vi "PropertyEditor.vi"(7 "Popup? (F)":bool, 8 "error in (no error)":errorcluster, 11 "Component in":refnum<class "IComponent.lvclass">) -> (0 "error out":errorcluster)   [LabVIEW 2022 SP3, in "Property Editor.lvlib"]
uses:
  <instrlib>/openDAQ/Examples/Property Editor/Property Editor.lvlib
  <instrlib>/openDAQ/Public/Classes/IComponent/IComponent.lvclass
  C:/Program Files (x86)/National Instruments/LabVIEW 2022/instr.lib/openDAQ/Public/Classes/IBaseObject/IBaseObject.lvclass
  C:/Program Files (x86)/National Instruments/LabVIEW 2022/instr.lib/openDAQ/Public/Classes/IPropertyObject/IPropertyObject.lvclass
  <instrlib>/openDAQ/Examples/Property Editor/TypeDef/State.ctl
  <instrlib>/openDAQ/Examples/Property Editor/TypeDef/Context.ctl
  <instrlib>/openDAQ/Public/Classes/IProperty/IProperty.lvclass
  <instrlib>/openDAQ/Examples/Property Editor/TypeDef/DisplayType.ctl
  <vilib>/picture/picture.llb/imagedata.ctl
  <vilib>/Utility/miscctls.llb/LVComboBoxStrsAndValuesArrayTypeDef.ctl
  <instrlib>/openDAQ/Public/Classes/IBaseObject/IBaseObject.lvclass/IBaseObject.ctl
  <instrlib>/openDAQ/Public/Classes/IBaseObject/Accessor/Read reference.vi
  <vilib>/Utility/error.llb/Trim Whitespace One-Sided.vi
  <instrlib>/openDAQ/Public/Classes/IInstance/IInstance.lvclass
  C:/Program Files (x86)/National Instruments/LabVIEW 2022/instr.lib/openDAQ/Public/Classes/IComponent/IComponent.lvclass
  <instrlib>/openDAQ/Public/Classes/IDevice/IDevice.lvclass
  <instrlib>/openDAQ/Public/Classes/daqCoreTypes/IFloat/IFloat.lvclass
  <instrlib>/openDAQ/Public/Classes/daqCoreTypes/IInteger/IInteger.lvclass
  <instrlib>/openDAQ/Public/Classes/daqCoreTypes/IBoolean/IBoolean.lvclass
  <instrlib>/openDAQ/Public/Classes/daqCoreTypes/IString/IString.lvclass
  <instrlib>/openDAQ/Public/Classes/daqCoreTypes/IRatio/IRatio.lvclass
  <instrlib>/openDAQ/Public/Classes/daqCoreTypes/IList/IList.lvclass
  <instrlib>/openDAQ/Public/Classes/IBaseObject/Polymorphic/borrowInterface/borrowListInterface.vi
  <instrlib>/openDAQ/Public/Classes/daqCoreTypes/IList/Polymorphic/getList/getStringList.vi
  <instrlib>/openDAQ/Public/Classes/daqCoreTypes/IList/Polymorphic/getList/getFloatList.vi
  <instrlib>/openDAQ/Public/Classes/daqCoreTypes/IList/Polymorphic/getList/getIntegerList.vi
  <instrlib>/openDAQ/Public/Classes/IBaseObject/Polymorphic/borrowInterface/borrowDictInterface.vi
  <instrlib>/openDAQ/Public/Classes/daqCoreTypes/IDict/Polymorphic/getValueList/getIntegerValueList.vi
  <instrlib>/openDAQ/Public/Classes/daqCoreTypes/IDict/Polymorphic/getValueList/getFloatValueList.vi
  <instrlib>/openDAQ/Public/Classes/daqCoreTypes/IDict/Polymorphic/getValueList/getStringValueList.vi
  <instrlib>/openDAQ/Public/Classes/IBaseObject/IBaseObject.lvclass
  <instrlib>/openDAQ/Public/Classes/daqUtils/daqUtils.lvlib
  <instrlib>/openDAQ/Public/Classes/daqCoreTypes/IDict/IDict.lvclass
panel:
  in  "btn:PropertyRefresh":bool
  in  "Btn:Stop":bool
  in  "RB:Selector":T1(radio)
  in  "Tree.Components":string(tree)="Devices"
  in  "Tree.Properties":string(tree)
  in  "Selection Values":string(combo)
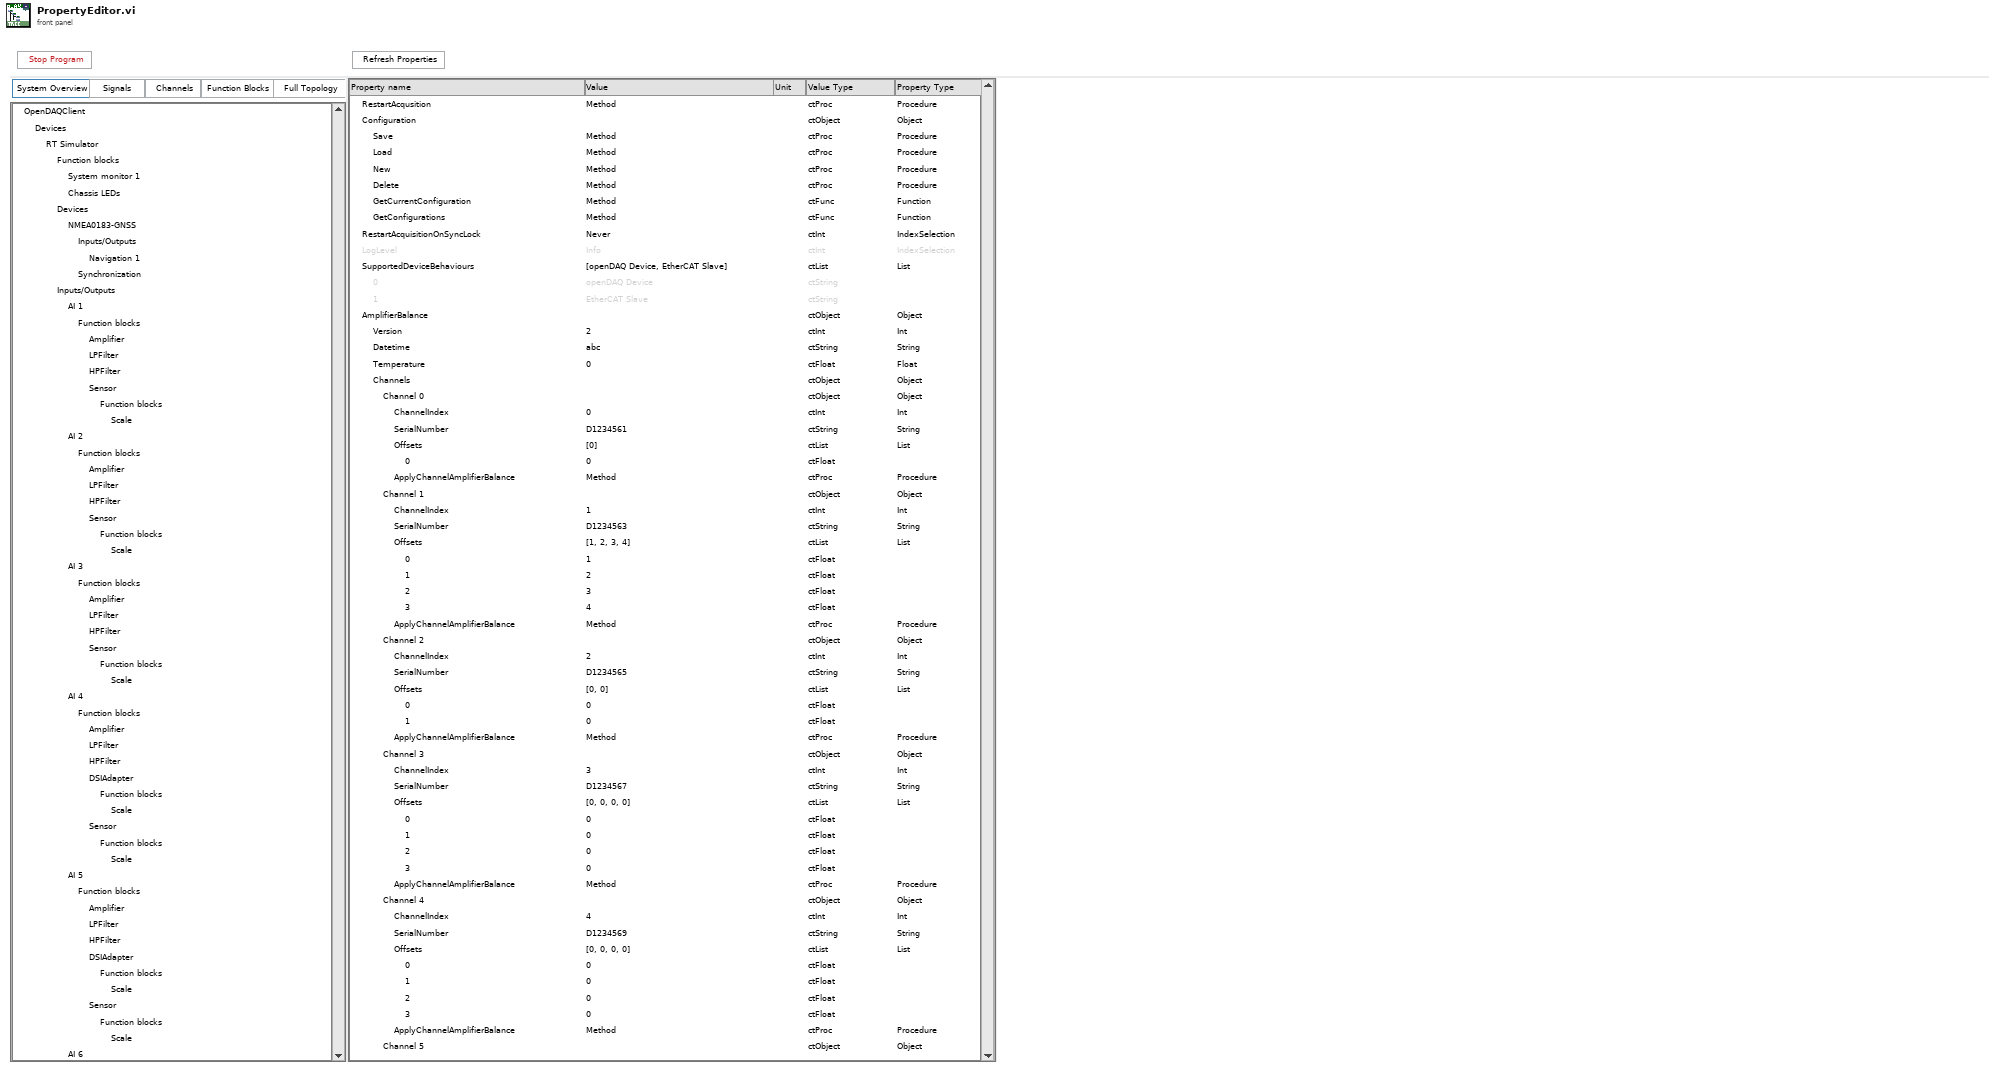
[diagram p1: front panel]
types:
  T1 = enum32{"Btn:SystemOverview", "Btn:Signals", "Btn:Channels", "Btn:FunctionBlocks", "Btn:FullTopology"}
  T2 = typedef "Property Editor.lvlib/Context.ctl" = cluster{"Simulator.Instance":refnum<class "IComponent.lvclass">, "Instance":refnum<class "IComponent.lvclass">, "Simulator":refnum<class "IComponent.lvclass">, "Nodes":map{string, refnum<class "IComponent.lvclass">}, "Selected.Node":refnum<class "IComponent.lvclass">, "Properties":map{string, refnum<class "IProperty.lvclass">}, "Selected.Property":refnum<class "IProperty.lvclass">, "Tree.Components.Ref":refnum<vi>, "Tree.Properties.Ref":refnum<vi>, "DisplayType":T3, "Readonly?":bool[]}
  T3 = typedef "Property Editor.lvlib/DisplayType.ctl" = enum16{"SYSTEM_OVERVIEW", "SIGNALS", "CHANNELS", "FUNCTION_BLOCKS", "TOPOLOGY", "TOPOLOGY_CUSTOM_COMPONENTS", "UNSPECIFIED"}
  T4 = typedef "Property Editor.lvlib/State.ctl" = enum16{"INIT", "- SIMULATOR.setup", "- COMPONENTS.traverse", "IDLE", "- PROPERTIES.traverse", "STOP", "ERROR"}
  T5 = typedef "LVComboBoxStrsAndValuesArrayTypeDef.ctl" = cluster{"String":string, "Value":string}[]
  T6 = typedef "imagedata.ctl" = cluster{"image type":i32, "image depth":i32, "image":u8[], "mask":u8[], "colors":u32[], "Rectangle":cluster{"left":i16, "top":i16, "right":i16, "bottom":i16}}
  T7 = typedef "LVPoint32TypeDef.ctl" = cluster{"Horizontal":i32, "Vertical":i32}
  T8 = typedef "openDAQ.lvlib/CoreType.ctl" = u16
  T9 = typedef "openDAQ.lvlib/PropertyType.ctl" = u16
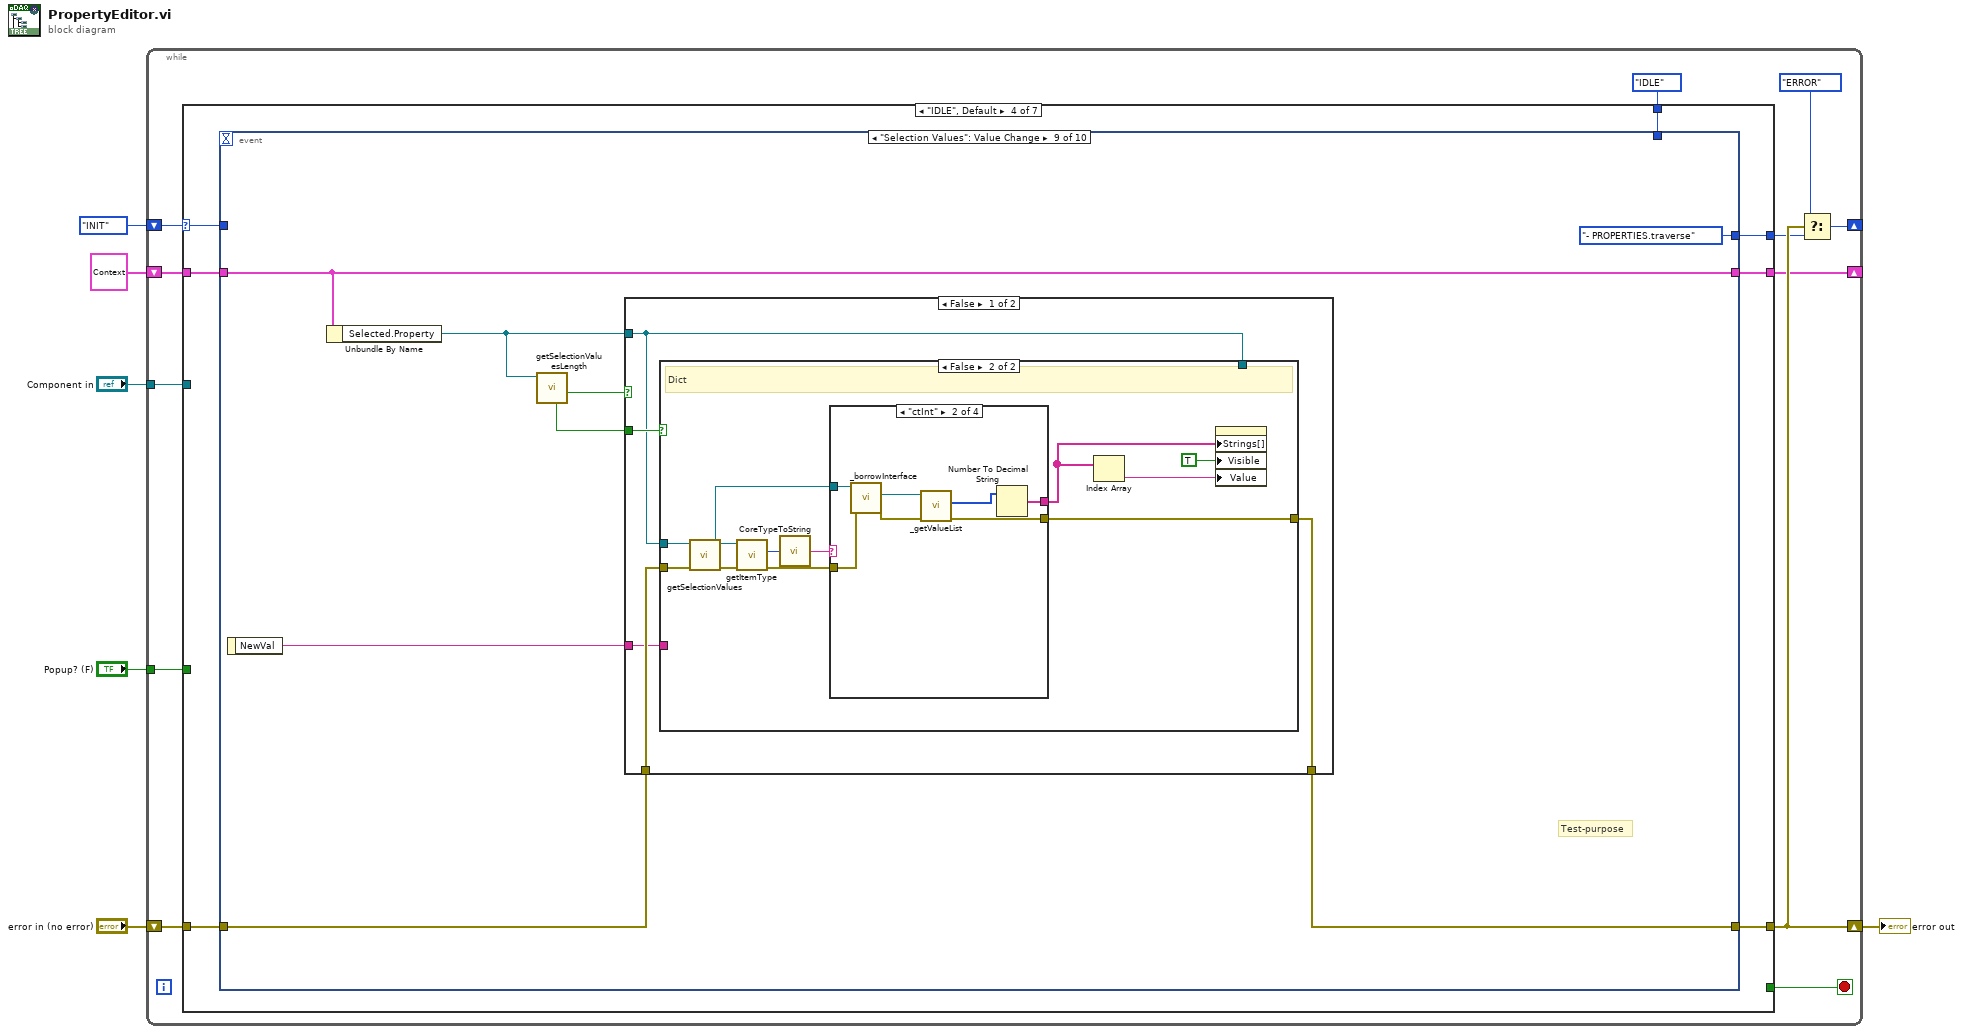
[diagram p0: block diagram]
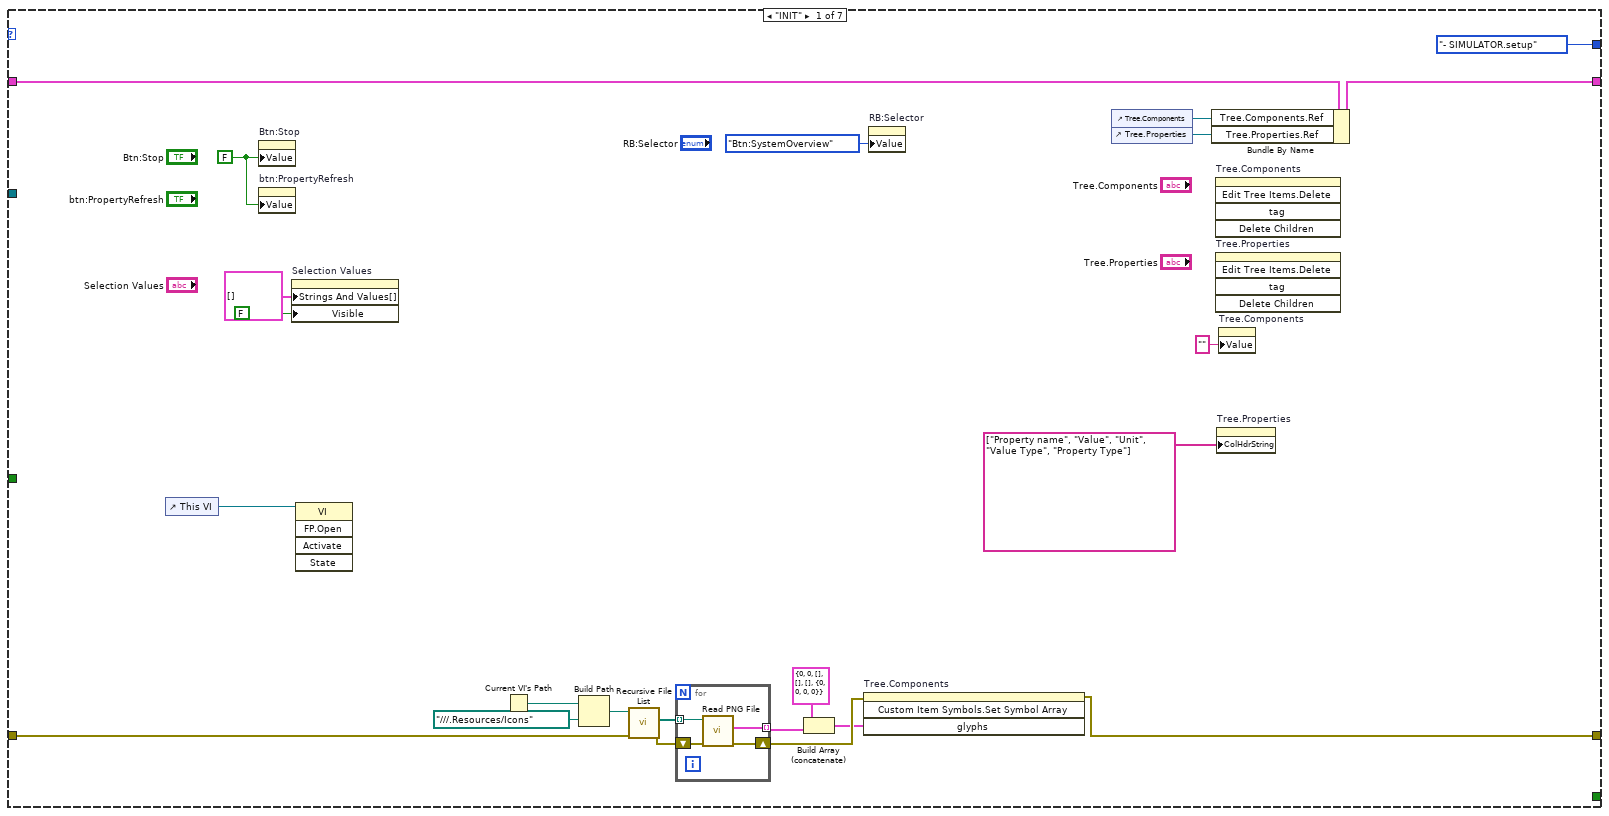
[diagram p2: hidden frame]
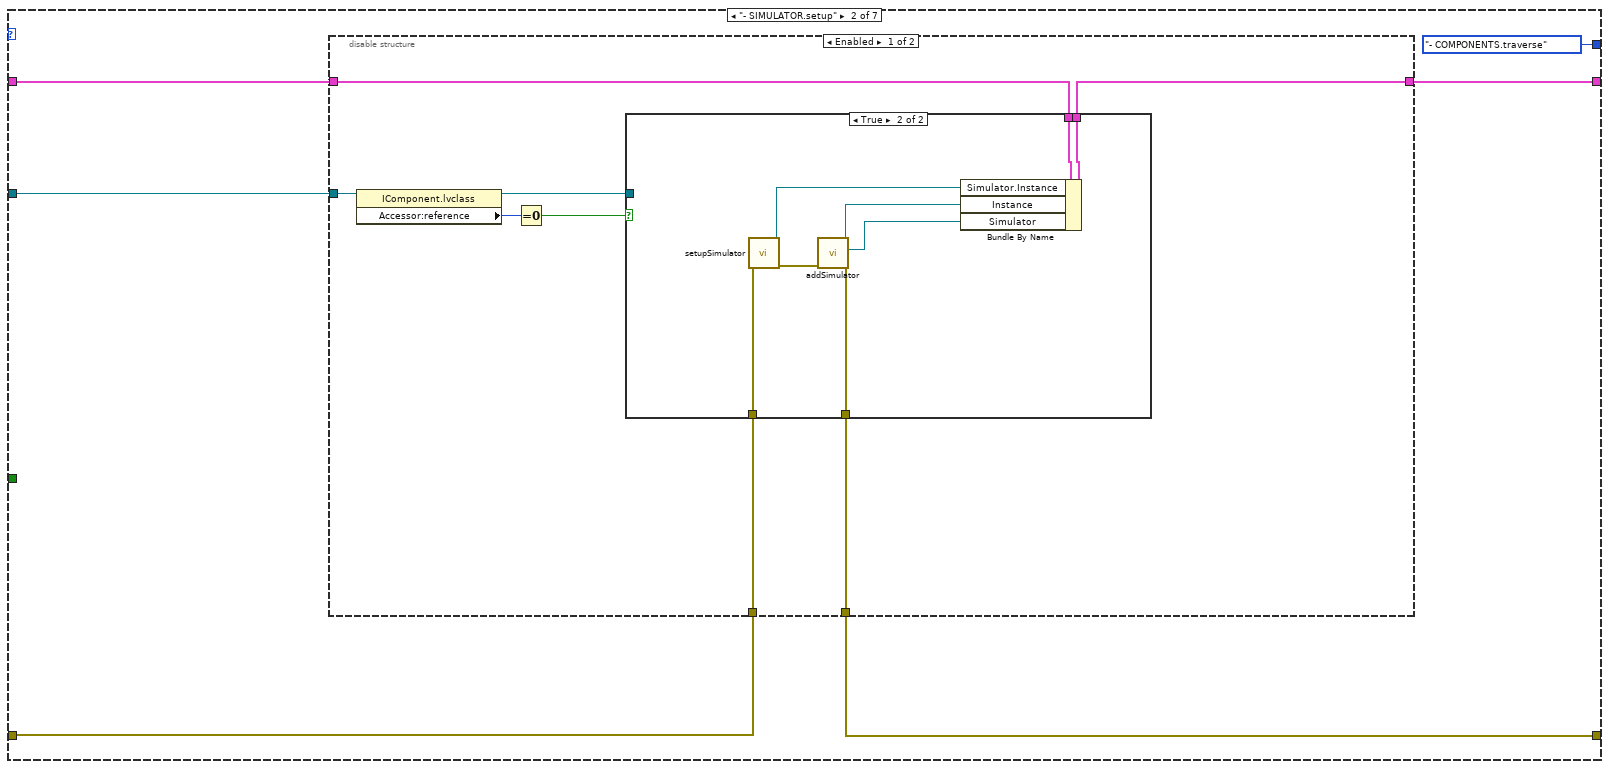
[diagram p3: hidden frame]
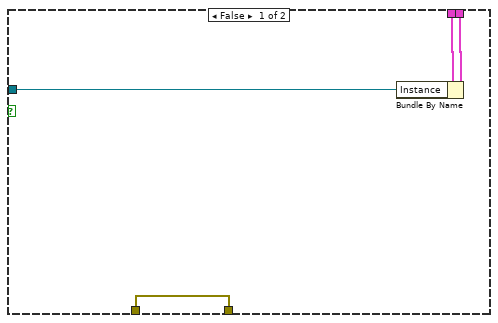
[diagram p4: hidden frame]
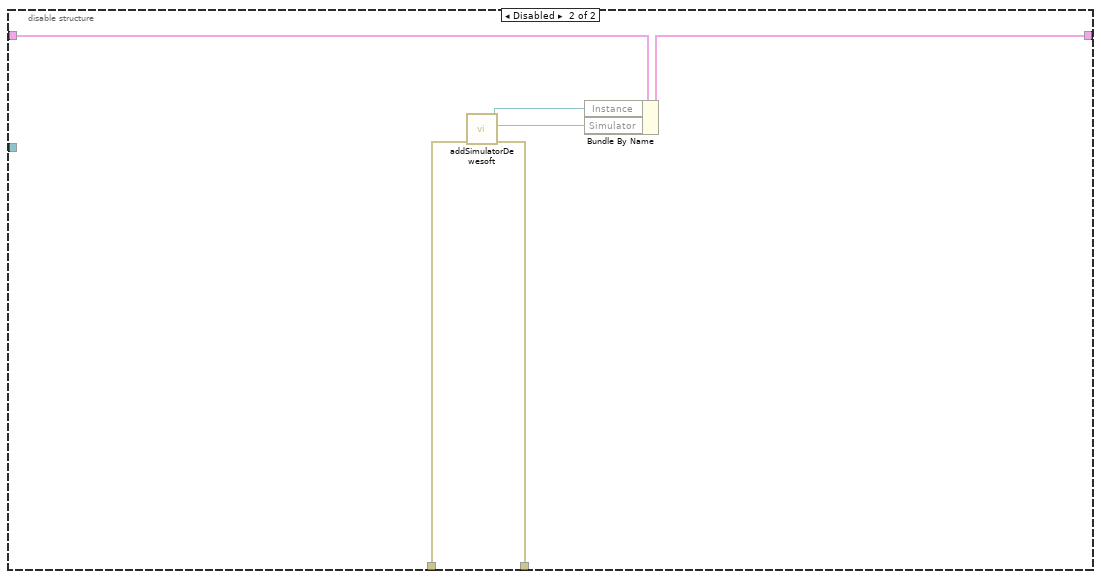
[diagram p5: hidden frame]
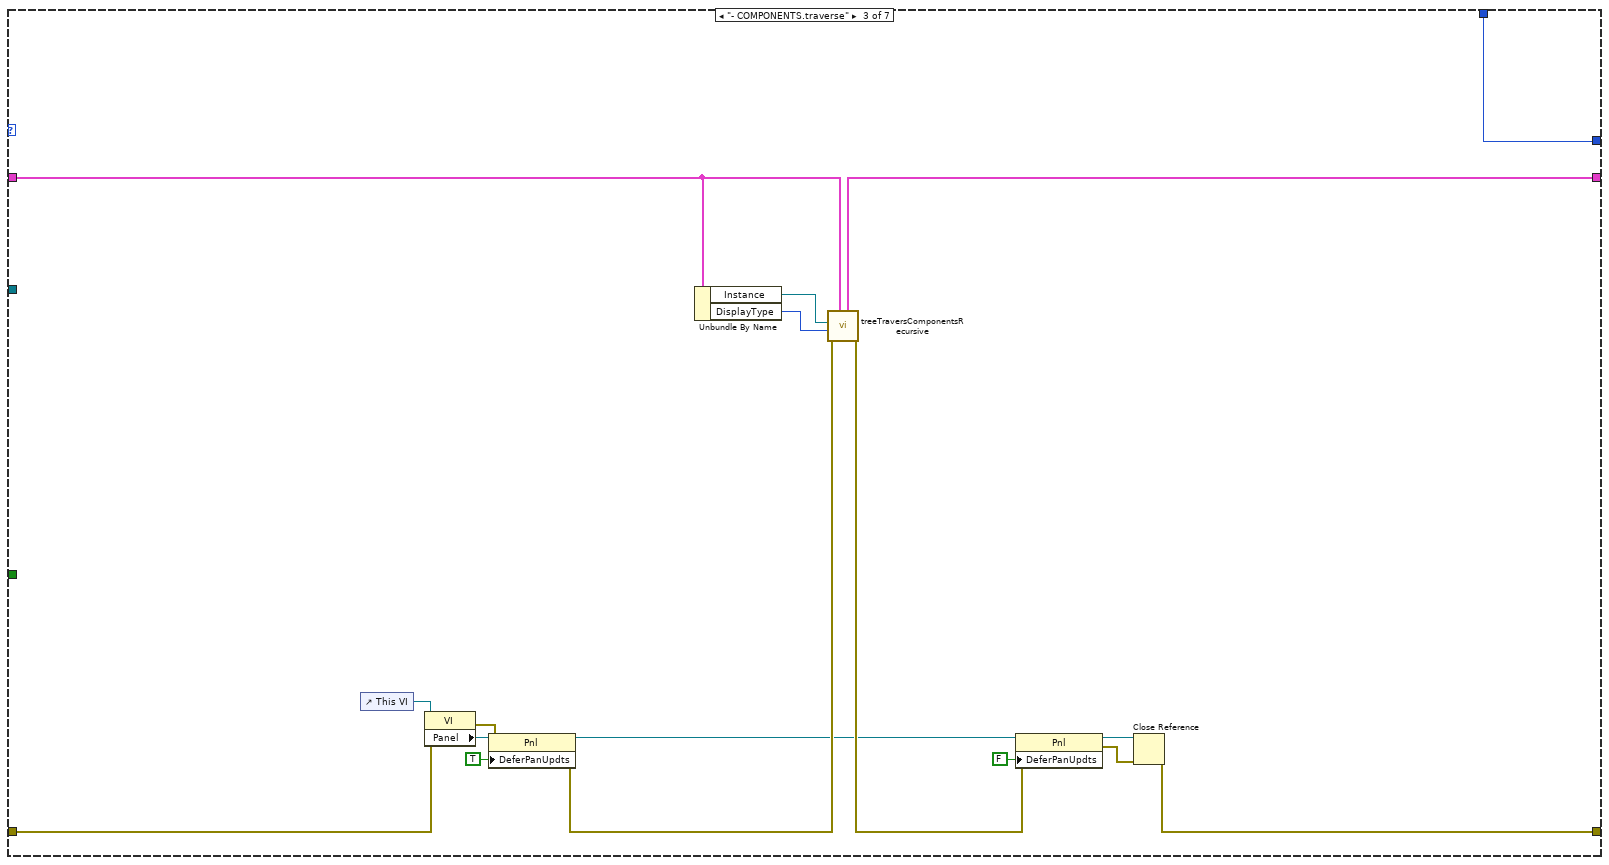
[diagram p6: hidden frame]
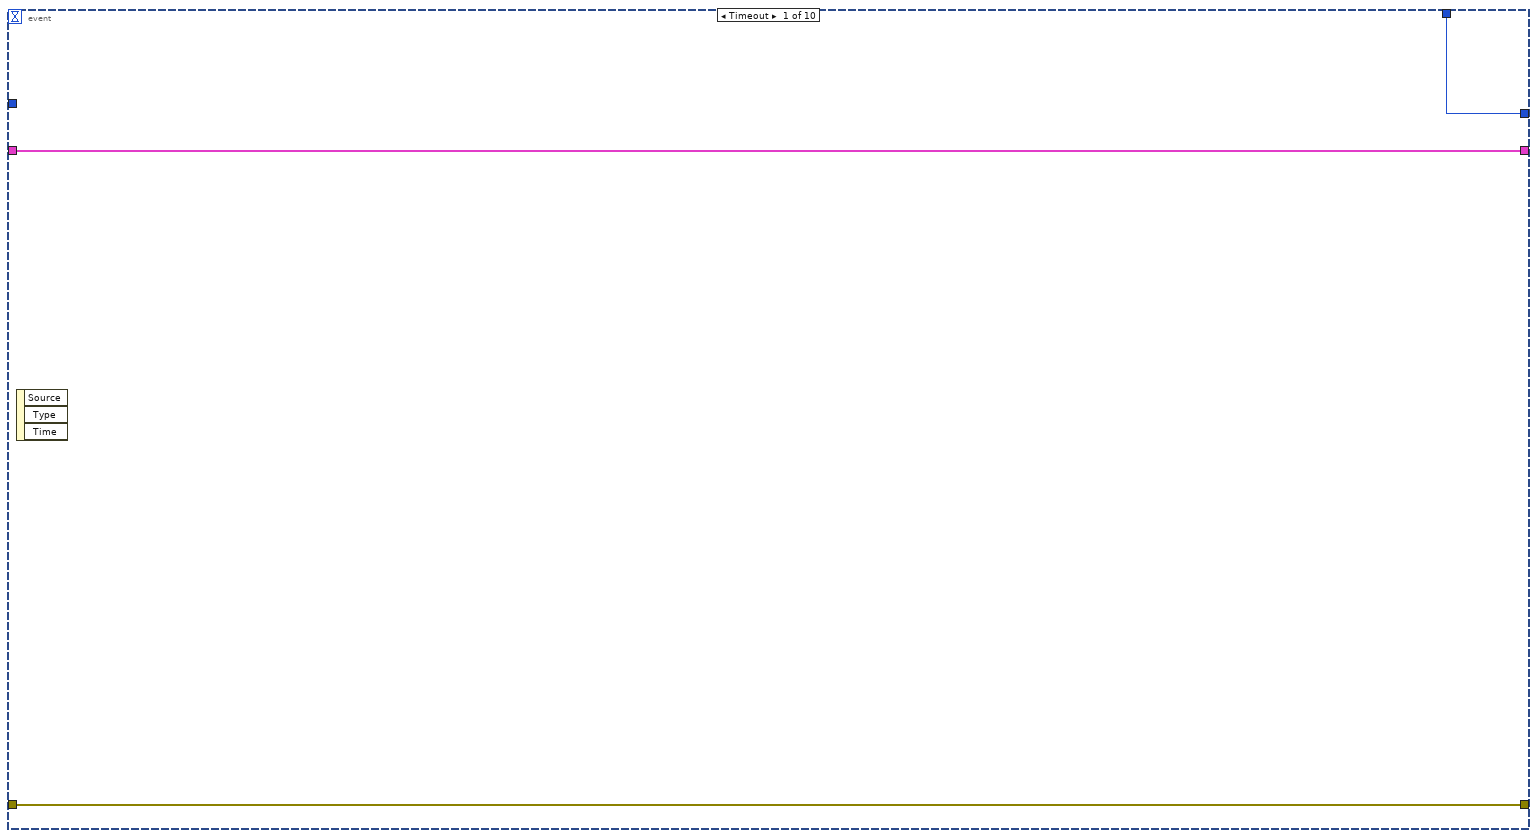
[diagram p7: hidden frame]
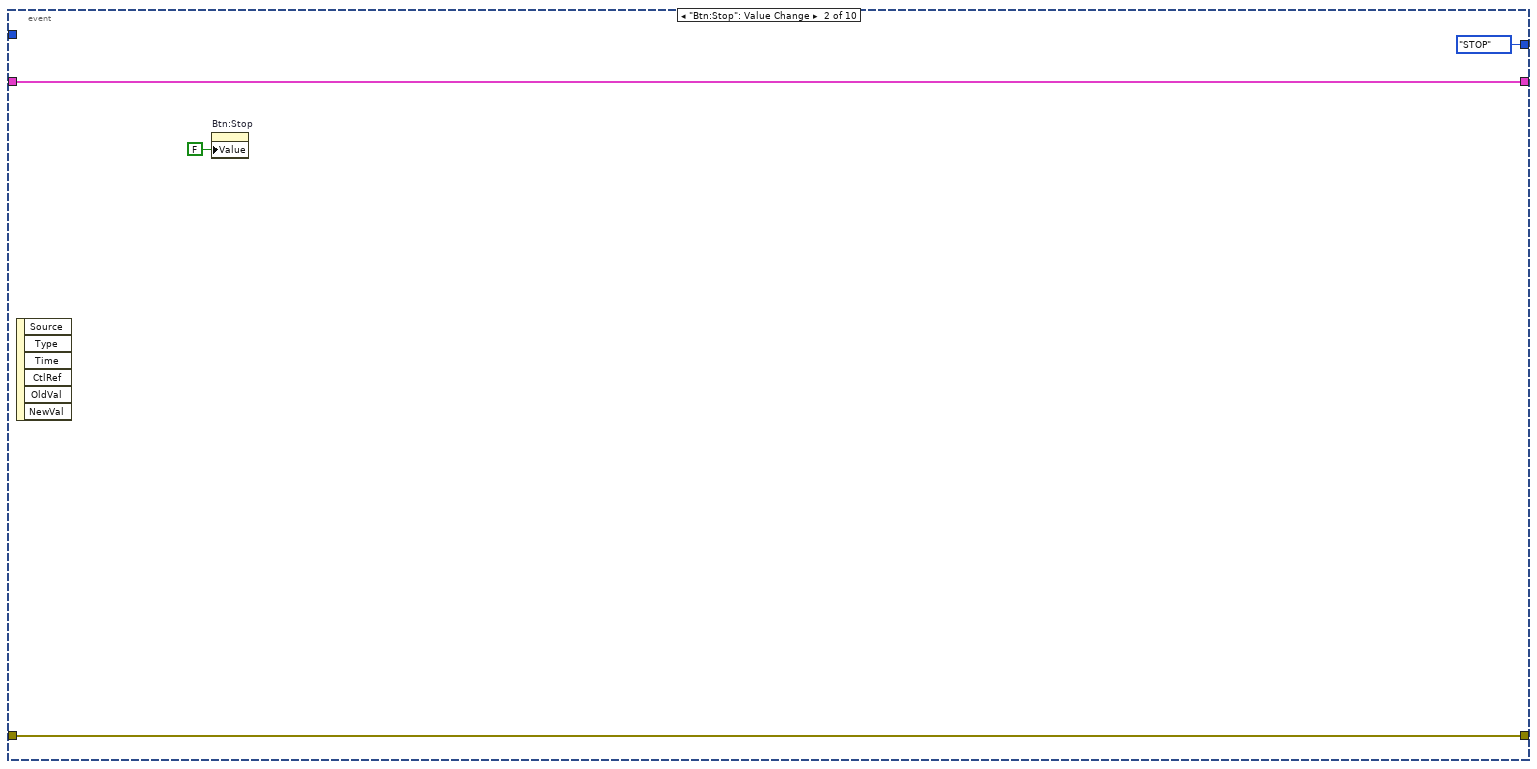
[diagram p8: hidden frame]
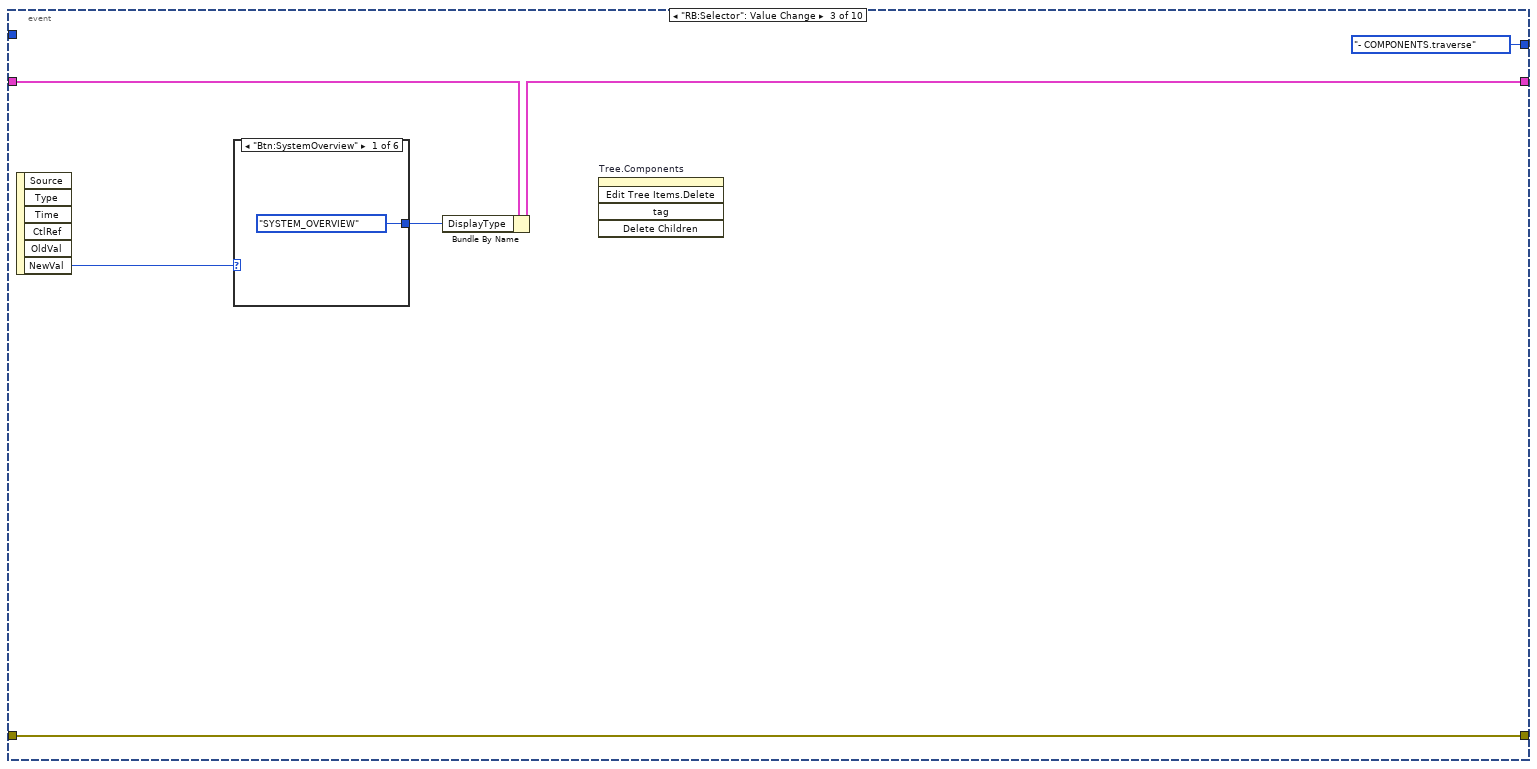
[diagram p9: hidden frame]
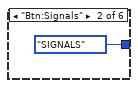
[diagram p10: hidden frame]
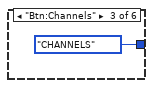
[diagram p11: hidden frame]
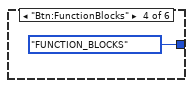
[diagram p12: hidden frame]
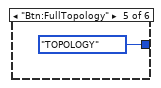
[diagram p13: hidden frame]
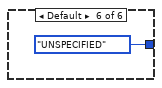
[diagram p14: hidden frame]
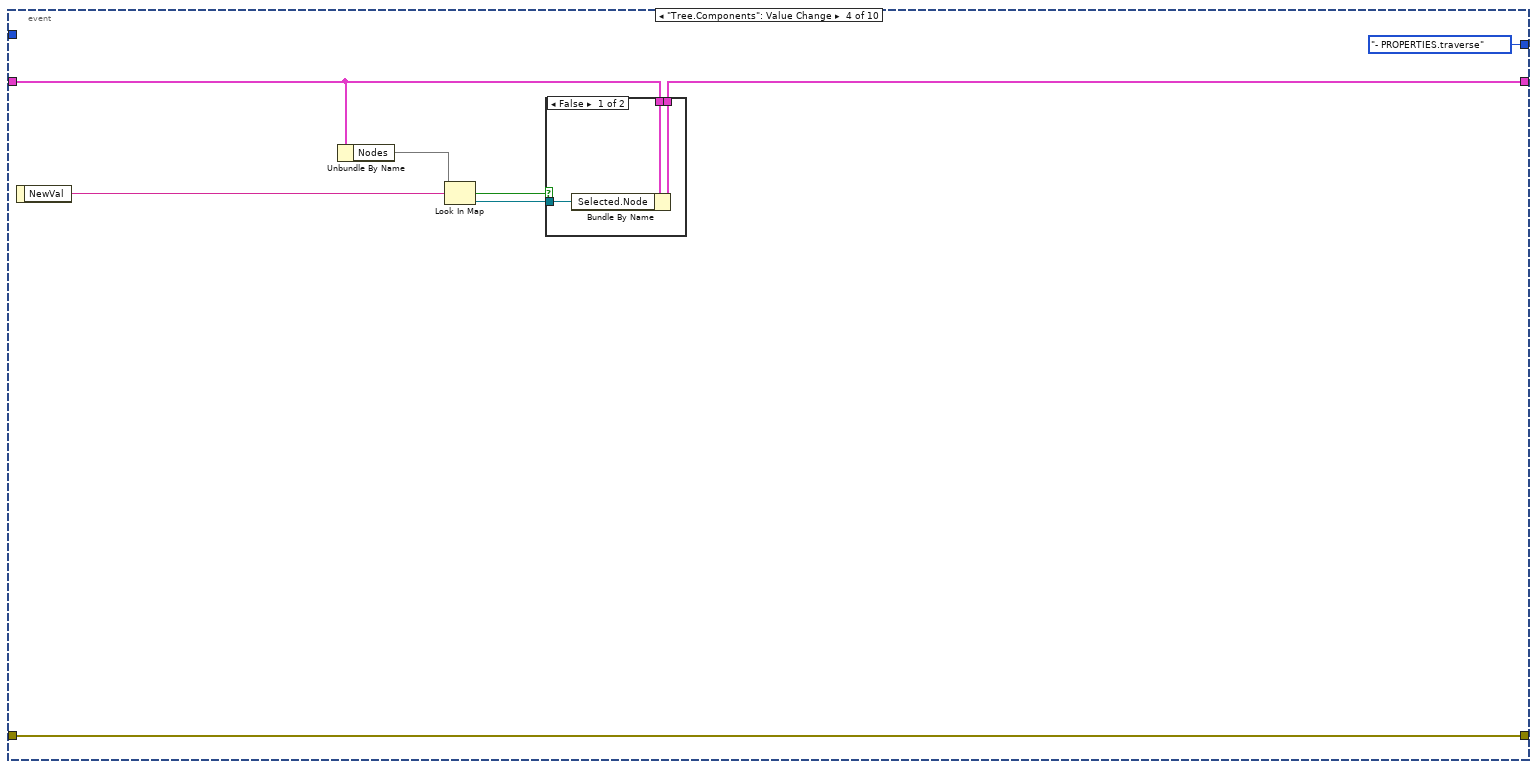
[diagram p15: hidden frame]
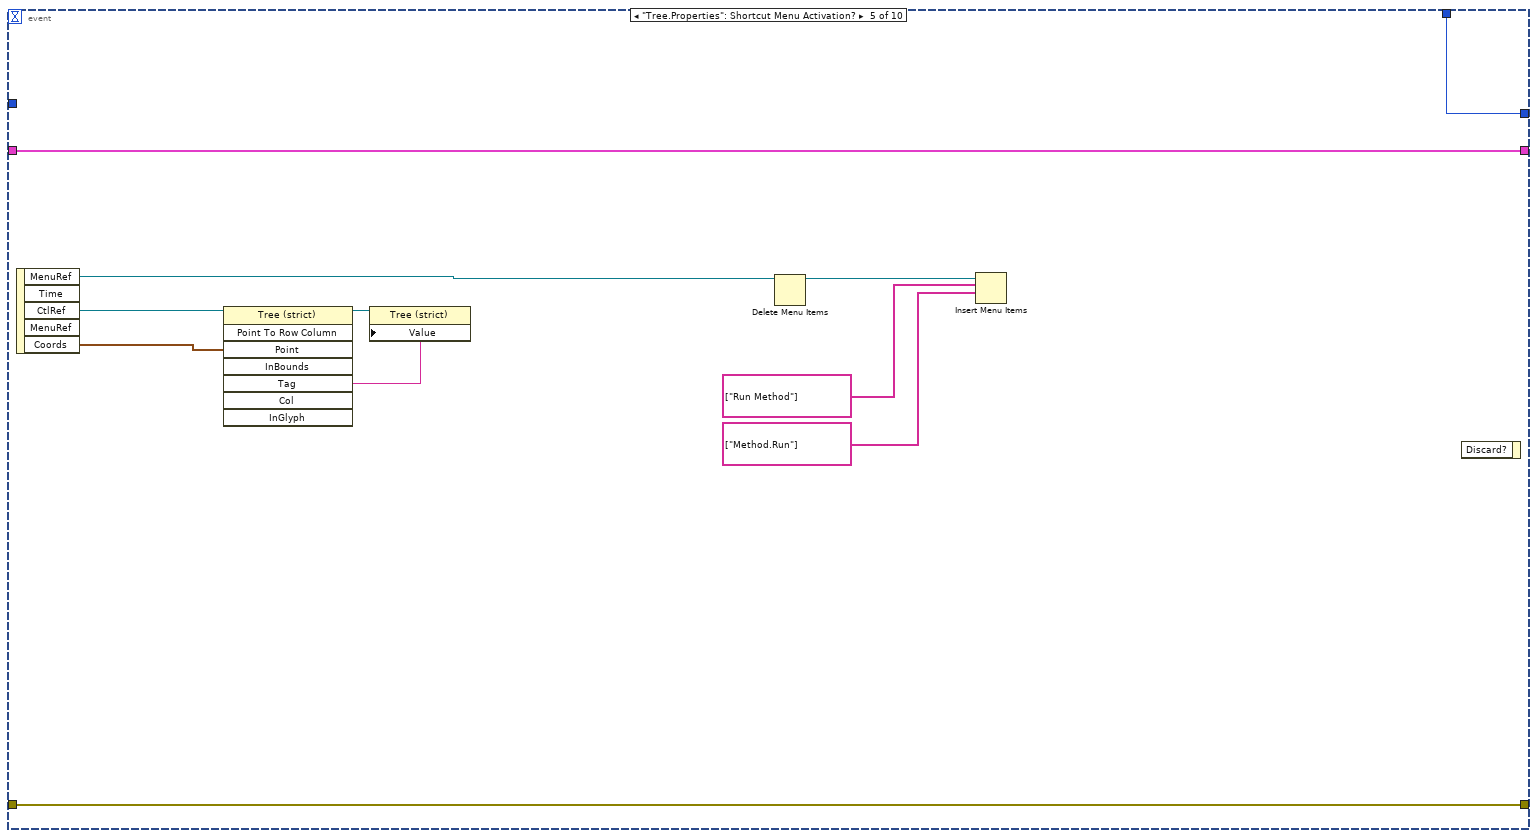
[diagram p17: hidden frame]
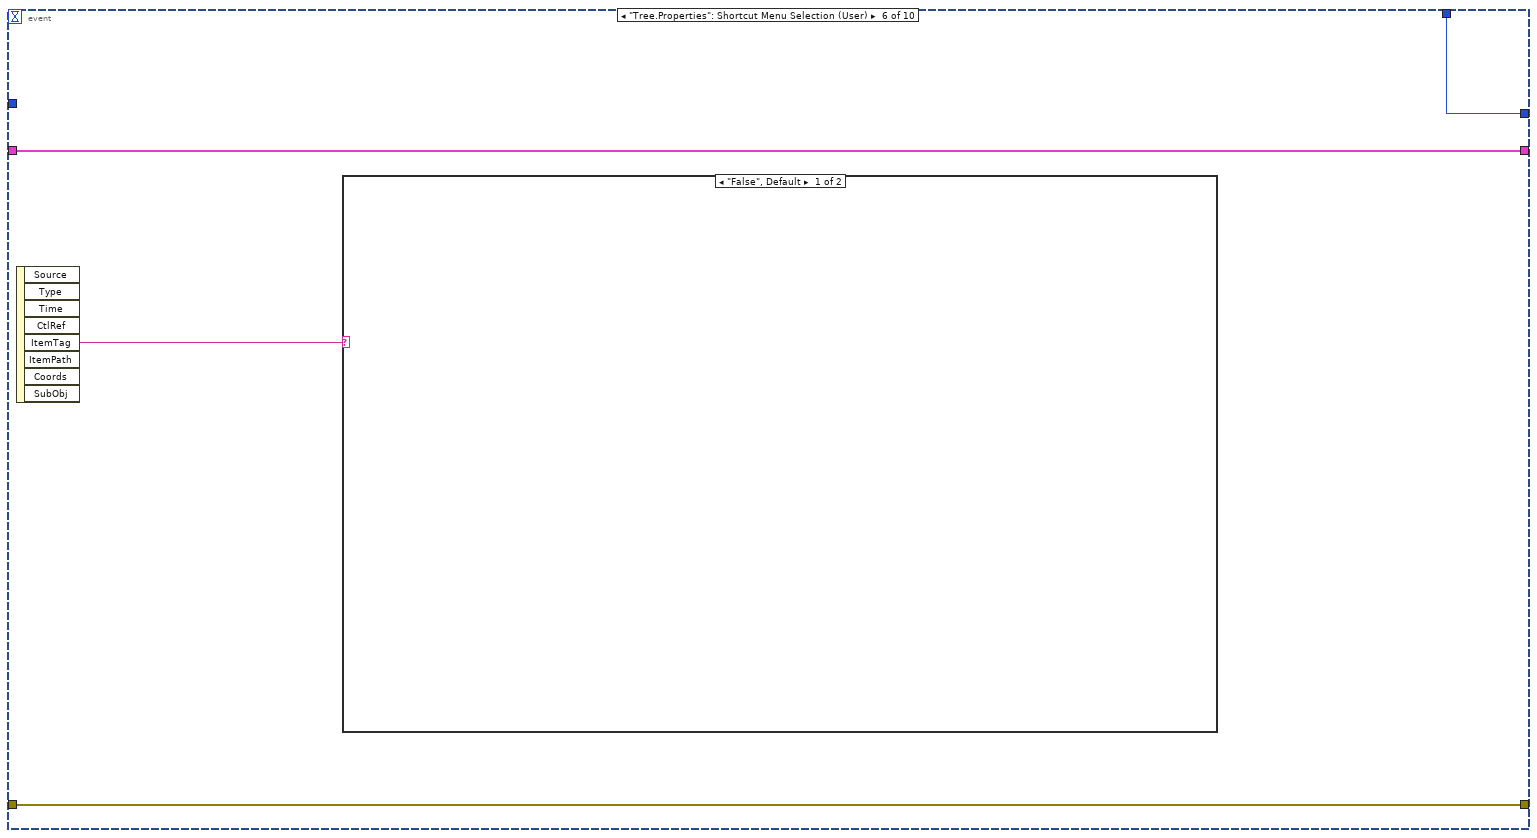
[diagram p18: hidden frame]
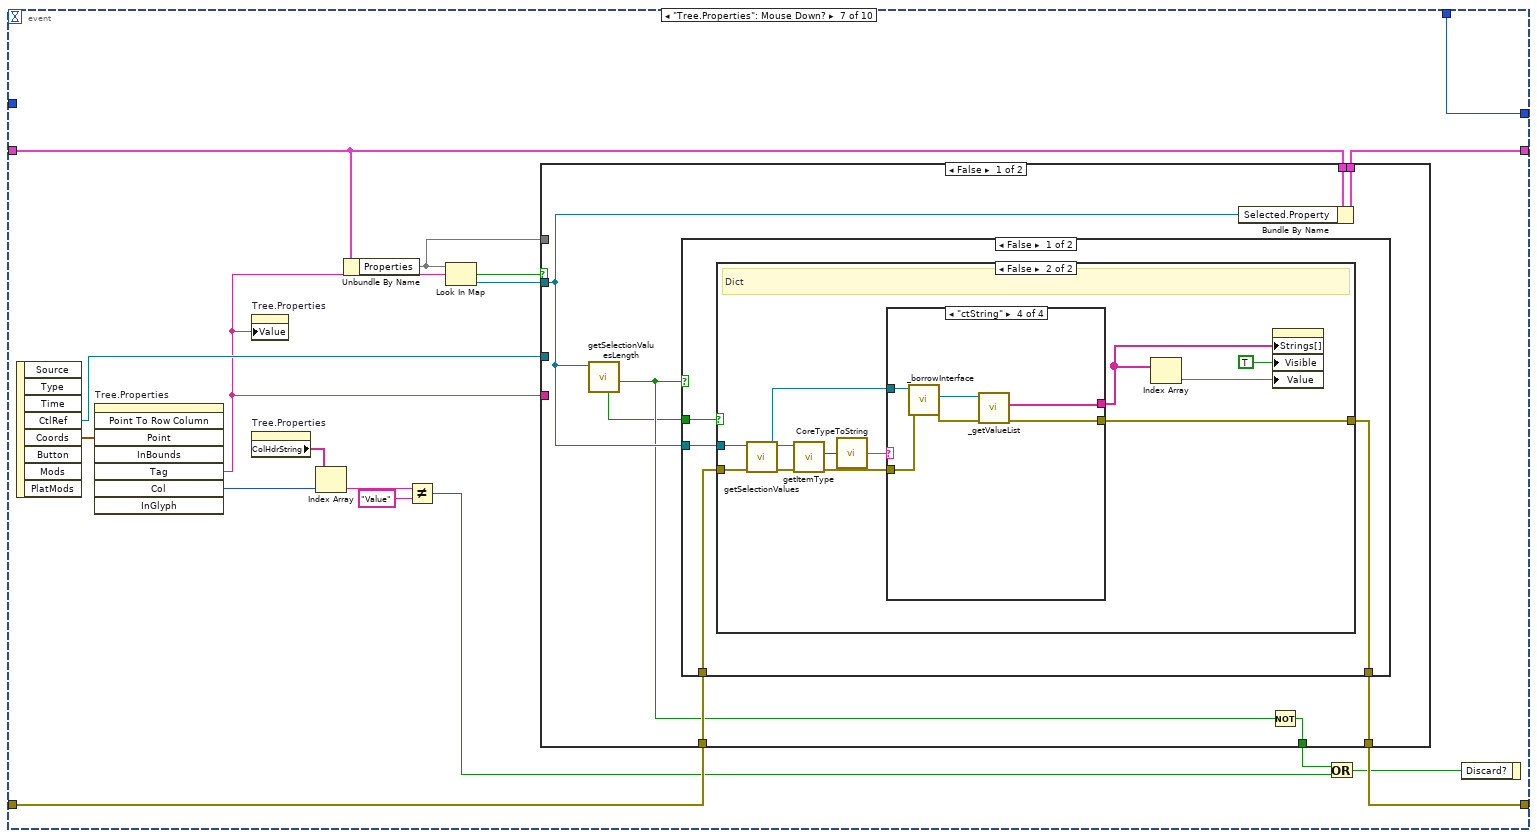
[diagram p20: hidden frame]
diagram:
  n1 = while {
    shift-right: [w15] -> _
    shift-left: State."INIT" ("Enum") -> [w17]
    shift-right: [w18] -> w2
    shift-left: "error in (no error)" -> [w14]
    shift-right: [w10] -> _
    shift-left: T2 {"Simulator.Instance"=refnum, "Instance"=refnum, "Simulator"=refnum, "Nodes"={}, "Selected.Node"=refnum, "Properties"={}, "Selected.Property"=refnum, "Tree.Components.Ref"=refnum, "Tree.Properties.Ref"=refnum, "DisplayType"=enum."SYSTEM_OVERVIEW", "Readonly?"=[]} -> [w11]
    tunnel: "Component in" -> [w8]
    tunnel: "Popup? (F)" -> [w7]
    stop <- w9 stop-if-true
    n2 = case shown="\"IDLE\", Default" w17 {
      selector: w17 -> [_ _ _ w101 _ _ _]
      tunnel: [State."- SIMULATOR.setup" ("Enum") State."- COMPONENTS.traverse" ("Enum") w94 w100 w518 w535 State."STOP" ("Enum")] -> w13
      tunnel: State."IDLE" ("Enum") -> [_ _ w94 w99 w518 w535 _]
      tunnel: w14 -> [w36 w51 w88 w95 w517 w536 w547]
      tunnel: [w28 w47 w82 w98 w516 w536 w546] -> w18
      tunnel: w11 -> [w31 w50 w93 w97 w513 w534 w544]
      tunnel: [w27 w49 w90 w96 w511 w534 w544] -> w10
      tunnel: [_ _ _ _ _ TRUE _] -> w9
      tunnel: w8 -> [_ w46 _ _ _ _ _]
      tunnel: w7 -> [_ _ _ _ _ w527 _]
      frame "INIT" {
        w20 = FALSE ("Btn:Stop")
        n3 = control-ref of="This VI"() -> (w19:refnum<vi>)
        n4 = property on="Btn:Stop" class="Bool (strict)"("Value"=w20) -> ()  [unwired: 2 in, 2 out]
        n5 = property on="btn:PropertyRefresh" class="Bool (strict)"("Value"=w20) -> ()  [unwired: 2 in, 2 out]
        n6 = property on="Selection Values" class="CmbBox"("Strings And Values[]"=T5 [] ("Strings And Values []"), "Visible"=FALSE) -> ()  [unwired: 2 in, 2 out]
        n7 = invoke class="VI" method="FP.Open"(reference=w19) -> ()  [unwired: 4 in, 5 out]
        n8 = Current VI's Path() -> (path=w39:path)
        n9 = Build Path(base path=w39, name or relative path=path "../../../.Resources/Icons") -> (appended path=w37:path)
        n10 = call <vilib>:"Recursive File List.vi"("error in (no error)"=w36, "Folder Path"=w37) -> ("error out"=w34:errorcluster, "All Files in Dir"=w35:path[])  [unwired: 5 in, 3 out]
        n11 = for {
          tunnel: w35 -> [w45] mode=indexing
          shift-right: [w43] -> w41
          shift-left: w34 -> [w44]
          tunnel: [w42] -> w32 mode=indexing
          n12 = call <vilib>:"Read PNG File.vi"("error in (no error)"=w44, "path to PNG file"=w45) -> ("error out"=w43:errorcluster, "image data"=w42:T6)  [unwired: 7 in, 1 out]
        }
        n13 = Build Array (concatenate)(T6 {"image type"=0, "image depth"=0, "image"=[], "mask"=[], "colors"=[], "Rectangle"={"left"=0, "top"=0, "right"=0, "bottom"=0}} ("image data"), w32) -> (w29:T6[])
        n14 = invoke on="Tree.Components" class="Tree (strict)" method="Custom Item Symbols.Set Symbol Array"(error in=w41, "glyphs"=w29) -> (error out=w28:errorcluster)  [unwired: 2 in, 3 out]
        n15 = property on="RB:Selector" class="RadioBtnsControl (strict)"("Value"=T1."Btn:SystemOverview" ("RB:Selector")) -> ()  [unwired: 2 in, 2 out]
        n16 = control-ref of="Tree.Components"() -> (w30:refnum<vi>)
        n17 = control-ref of="Tree.Properties"() -> (w23:refnum<vi>)
        n18 = Bundle By Name(cluster=w31, "Tree.Components.Ref"=w30, "Tree.Properties.Ref"=w23) -> (w27:T2)
        n19 = invoke on="Tree.Components" class="Tree (strict)" method="Edit Tree Items.Delete"() -> ()  [unwired: 5 in, 5 out]
        n20 = invoke on="Tree.Properties" class="Tree (strict)" method="Edit Tree Items.Delete"() -> ()  [unwired: 5 in, 5 out]
        n21 = property on="Tree.Properties" class="Tree (strict)"("ColHdrString"=string[] ["Property name", "Value", "Unit", "Value Type", "Property Type"] ("Column Header Strings[]")) -> ()  [unwired: 2 in, 2 out]
        n22 = property on="Tree.Components" class="Tree (strict)"("Value"="" ("Tree.View")) -> ()  [unwired: 2 in, 2 out]
      }
      frame "- SIMULATOR.setup" {
        n23 = disable-structure shown="Enabled" {
          disable-tunnel: w51 -> [w59 w77]
          disable-tunnel: w50 -> [w58 w76]
          disable-tunnel: [w57 w75] -> w49
          disable-tunnel: [w56 w73] -> w47
          disable-tunnel: w46 -> [w55 _]
          frame Enabled {
            n24 = property class="IComponent.lvclass"(reference=w55) -> (reference out=w52:refnum<class "IComponent.lvclass">, "Accessor:reference"=w54:i64)  [unwired: 1 in, 1 out]
            n25 = Equal To 0?(x=w54) -> (x = 0?=w53:bool)
            n26 = case shown="True" w53 {
              tunnel: w59 -> [w60 w71]
              tunnel: w58 -> [w63 w69]
              tunnel: [w61 w68] -> w57
              tunnel: [w60 w66] -> w56
              tunnel: w52 -> [w62 _]
              frame False {
                n27 = Bundle By Name(cluster=w63, "Instance"=w62) -> (w61:T2)
              }
              frame True {
                n28 = call <instrlib>:"setupSimulator.vi"("error in (no error)"=w71) -> ("error out"=w70:errorcluster, "IInstance out"=w64:refnum<class "IInstance.lvclass">)  [unwired: 9 in]
                n29 = call <instrlib>:"addSimulator.vi"("error in (no error)"=w70) -> ("error out"=w66:errorcluster, "IDevice out"=w67:refnum<class "IDevice.lvclass">, "IInstance out"=w65:refnum<class "IInstance.lvclass">)  [unwired: 8 in]
                n30 = Bundle By Name(cluster=w69, "Simulator.Instance"=w64, "Instance"=w65, "Simulator"=w67) -> (w68:T2)
              }
            }
          }
          frame Disabled {
            n31 = call <instrlib>:"addSimulatorDewesoft.vi"("error in (no error)"=w77) -> ("error out"=w73:errorcluster, "IDevice out"=w72:refnum<class "IDevice.lvclass">, "IInstance out"=w74:refnum<class "IInstance.lvclass">)  [unwired: 8 in]
            n32 = Bundle By Name(cluster=w76, "Instance"=w74, "Simulator"=w72) -> (w75:T2)
          }
        }
      }
      frame "- COMPONENTS.traverse" {
        n33 = control-ref of="This VI"() -> (w80:refnum<vi>)
        n34 = property class="VI"(reference=w80, error in=w88) -> (error out=w78:errorcluster, "Panel"=w79:refnum<vi>)  [unwired: 1 out]
        n35 = property class="Pnl"(reference=w79, error in=w78, "DeferPanUpdts"=TRUE ("Defer Panel Updates")) -> (reference out=w85:refnum<vi>, error out=w91:errorcluster)
        n36 = Unbundle By Name(w93) -> ("Instance"=w92:refnum<class "IComponent.lvclass">, "DisplayType"=w89:T3)
        n37 = call <instrlib>:"treeTraversComponentsRecursive.vi"("Cluster in"=w93, "error in (no error)"=w91, "DisplayType"=w89, "Component"=w92) -> ("error out"=w87:errorcluster, "Cluster out"=w90:T2)  [unwired: 6 in]
        n38 = property class="Pnl"(reference=w85, error in=w87, "DeferPanUpdts"=FALSE ("Defer Panel Updates")) -> (reference out=w84:refnum<vi>, error out=w83:errorcluster)
        n39 = Close Reference(reference=w84, error in (no error)=w83) -> (error out=w82:errorcluster)
      }
      frame "IDLE", Default {
        n40 = event shown="[8] \"Selection Values\": Value Change" {
          selector: _ -> [_ _ _ _ _ _ _ _ _ _]
          dyn-events: _ -> [_ _ _ _ _ _ _ _ _ _]
          timeout: _ -> [_ _ _ _ _ _ _ _ _ _]
          tunnel: w101 -> [_ _ _ _ _ _ _ _ _ _]
          tunnel: [w104 State."STOP" ("Enum") State."- COMPONENTS.traverse" ("Enum") State."- PROPERTIES.traverse" ("Enum") w140 w146 w161 State."- PROPERTIES.traverse" ("Enum") State."- PROPERTIES.traverse" ("Enum") State."- PROPERTIES.traverse" ("Enum")] -> w100
          tunnel: w99 -> [w104 _ _ _ w140 w146 w161 _ _ _]
          tunnel: [w103 w105 w113 w124 w138 w144 w165 w287 w389 w497] -> w98
          tunnel: w95 -> [w103 w105 w113 w124 w138 w144 w157 w280 w395 w497]
          tunnel: w97 -> [w102 w108 w112 w122 w139 w145 w152 w289 w392 w499]
          tunnel: [w102 w108 w111 w123 w139 w145 w153 w289 w392 w499] -> w96
          event Timeout {
            n41 = event-data() -> ()  [unwired: 1 in, 3 out]
          }
          event "Btn:Stop": Value Change {
            n42 = event-data() -> ()  [unwired: 1 in, 6 out]
            n43 = property on="Btn:Stop" class="Bool (strict)"("Value"=FALSE ("Btn:Stop")) -> ()  [unwired: 2 in, 2 out]
          }
          event "RB:Selector": Value Change {
            n44 = event-data() -> ("NewVal"=w114:T1)  [unwired: 1 in, 5 out]
            n45 = case shown="\"Btn:SystemOverview\"" w114 {
              tunnel: [DisplayType."SYSTEM_OVERVIEW" ("DisplayType") DisplayType."SIGNALS" ("DisplayType") DisplayType."CHANNELS" ("DisplayType") DisplayType."FUNCTION_BLOCKS" ("DisplayType") DisplayType."TOPOLOGY" ("DisplayType") DisplayType."UNSPECIFIED" ("DisplayType")] -> w110
              frame "Btn:SystemOverview" {
              }
              frame "Btn:Signals" {
              }
              frame "Btn:Channels" {
              }
              frame "Btn:FunctionBlocks" {
              }
              frame "Btn:FullTopology" {
              }
              frame Default {
              }
            }
            n46 = Bundle By Name(cluster=w112, "DisplayType"=w110) -> (w111:T2)
            n47 = invoke on="Tree.Components" class="Tree (strict)" method="Edit Tree Items.Delete"() -> ()  [unwired: 5 in, 5 out]
          }
          event "Tree.Components": Value Change {
            n48 = event-data() -> ("NewVal"=w127:string)  [unwired: 1 in]
            n49 = Unbundle By Name(w122) -> ("Nodes"=w128:map{string, refnum<class "IComponent.lvclass">})
            n50 = Look In Map(map=w128, key=w127) -> (key not found?=w126:bool, value=w125:refnum<class "IComponent.lvclass">)  [unwired: 1 in]
            n51 = case shown="False" w126 {
              tunnel: w125 -> [w130 _]
              tunnel: w122 -> [w131 w132]
              tunnel: [w129 w132] -> w123
              frame False {
                n52 = Bundle By Name(cluster=w131, "Selected.Node"=w130) -> (w129:T2)
              }
              frame True {
              }
            }
          }
          event "Tree.Properties": Shortcut Menu Activation? {
            n53 = event-data() -> ("MenuRef"=w136:refnum<k9>, "CtlRef"=w143:refnum<vi>, "Coords"=w142:T7)  [unwired: 1 in, 2 out]
            n54 = invoke class="Tree (strict)" method="Point To Row Column"(reference=w143, "Point"=w142) -> (reference out=w141:refnum<vi>, "Tag"=w137:string)  [unwired: 6 in, 6 out]
            n55 = property class="Tree (strict)"(reference=w141, "Value"=w137) -> ()  [unwired: 1 in, 2 out]
            n56 = Delete Menu Items(9:w136) -> (3:w135:refnum<k9>)  [unwired: 3 in, 1 out]
            n57 = Insert Menu Items(7:string[] ["Method.Run"], 8:string[] ["Run Method"], 9:w135) -> ()  [unwired: 3 in, 3 out]
            n58 = event-data() -> ()  [unwired: 2 in, 1 out]
          }
          event "Tree.Properties": Shortcut Menu Selection (User) {
            n59 = event-data() -> ("ItemTag"=w147:string)  [unwired: 1 in, 7 out]
            n60 = case shown="\"False\", Default" w147 {
              frame "False", Default {
              }
              frame "Method.Run" {
              }
            }
          }
          event "Tree.Properties": Mouse Down? {
            n61 = event-data() -> ("CtlRef"=w149:refnum<vi>, "Coords"=w160:T7)  [unwired: 1 in, 6 out]
            n62 = invoke on="Tree.Properties" class="Tree (strict)" method="Point To Row Column"("Point"=w160) -> ("Tag"=w148:string, "Col"=w159:i32)  [unwired: 7 in, 6 out]
            n63 = property on="Tree.Properties" class="Tree (strict)"("Value"=w148) -> ()  [unwired: 2 in, 2 out]
            n64 = property on="Tree.Properties" class="Tree (strict)"() -> ("ColHdrString"=w164:string[])  [unwired: 2 in, 2 out]
            n65 = Index Array(array=w164, index=w159) -> (element=w163:string)
            n66 = Unbundle By Name(w152) -> ("Properties"=w150:map{string, refnum<class "IProperty.lvclass">})
            n67 = Not Equal?(x=w163, y="Value") -> (x != y?=w155:bool)
            n68 = Look In Map(map=w150, key=w148) -> (key not found?=w151:bool, value=w158:refnum<class "IProperty.lvclass">)  [unwired: 1 in]
            n69 = case shown="False" w151 {
              tunnel: [w173 w247] -> w165
              tunnel: w158 -> [w169 _]
              tunnel: w157 -> [w172 w257]
              tunnel: [w171 w248] -> w156
              tunnel: [w166 w249] -> w153
              tunnel: w152 -> [w170 w250]
              tunnel: w150 -> [_ w255]
              tunnel: w149 -> [_ w254]
              tunnel: w148 -> [_ w253]
              frame False {
                n70 = call <instrlib>:"getSelectionValuesLength.vi"("IProperty in"=w169) -> ("Selection Values Null?"=w168:bool, "List?"=w167:bool)  [unwired: 5 in, 4 out]
                n71 = case shown="False" w168 {
                  tunnel: [w175 w246] -> w173
                  tunnel: w169 -> [w174 _]
                  tunnel: w172 -> [w177 w246]
                  tunnel: w167 -> [w176 _]
                  frame False {
                    n72 = case shown="False" w176 {
                      tunnel: w174 -> [w189 w222]
                      tunnel: w177 -> [w188 w221]
                      tunnel: [w181 w214] -> w175
                      frame True {
                        # "List"
                        n73 = call <instrlib>:"getSelectionValues.vi"("error in (no error)"=w188, "IProperty in"=w189) -> ("error out"=w186:errorcluster, "Selection Values out"=w185:refnum<class "IBaseObject.lvclass">, "IProperty out"=w187:refnum<class "IProperty.lvclass">)  [unwired: 6 in, 1 out]
                        n74 = call <instrlib>:"getItemType.vi"("error in (no error)"=w186, "IProperty in"=w187) -> ("error out"=w182:errorcluster, "Item Type out"=w184:T8)  [unwired: 7 in, 1 out]
                        n75 = call <instrlib>:"CoreTypeToString.vi"("Value Type out"=w184) -> ("String"=w183:string)  [unwired: 4 in]
                        n76 = case shown="\"ctString\"" w183 {
                          tunnel: w185 -> [_ w194 w201 w208]
                          tunnel: w182 -> [w190 w193 w200 w207]
                          tunnel: [_ w192 w197 w204] -> w179
                          tunnel: [w190 w191 w199 w206] -> w181
                          frame Default {
                          }
                          frame "ctString" {
                            n77 = call-poly <instrlib>:"_borrowInterface.vi"("error in (no error)"=w193, "IBaseObject in"=w194) -> ("error out"=w195:errorcluster, "List out"=w196:refnum<class "IList.lvclass">)  [unwired: 6 in, 2 out]
                            n78 = call-poly <instrlib>:"_getList.vi"("error in (no error)"=w195, "IList in"=w196) -> ("error out"=w191:errorcluster, "String List out"=w192:string[])  [unwired: 8 in]
                          }
                          frame "ctFloat" {
                            n79 = call-poly <instrlib>:"_borrowInterface.vi"("error in (no error)"=w200, "IBaseObject in"=w201) -> ("error out"=w202:errorcluster, "List out"=w203:refnum<class "IList.lvclass">)  [unwired: 6 in, 2 out]
                            n80 = call-poly <instrlib>:"_getList.vi"("error in (no error)"=w202, "IList in"=w203) -> ("error out"=w199:errorcluster, "Floats out"=w198:dbl[])  [unwired: 8 in]
                            n81 = Number To Fractional String(number=w198) -> (F-format string=w197:string[])  [unwired: 3 in]
                          }
                          frame "ctInt" {
                            n82 = call-poly <instrlib>:"_borrowInterface.vi"("error in (no error)"=w207, "IBaseObject in"=w208) -> ("error out"=w209:errorcluster, "List out"=w210:refnum<class "IList.lvclass">)  [unwired: 6 in, 2 out]
                            n83 = call-poly <instrlib>:"_getList.vi"("error in (no error)"=w209, "IList in"=w210) -> ("error out"=w206:errorcluster, "Integers out"=w205:i32[])  [unwired: 8 in]
                            n84 = Number To Decimal String(number=w205) -> (decimal integer string=w204:string[])  [unwired: 1 in]
                          }
                        }
                        n85 = Index Array(array=w179) -> (element=w178:string)  [unwired: 1 in]
                        n86 = property on="Selection Values" class="CmbBox"("Strings[]"=w179, "Visible"=TRUE, "Value"=w178) -> ()  [unwired: 2 in, 2 out]
                      }
                      frame False {
                        # "Dict"
                        n87 = call <instrlib>:"getSelectionValues.vi"("error in (no error)"=w221, "IProperty in"=w222) -> ("error out"=w219:errorcluster, "Selection Values out"=w218:refnum<class "IBaseObject.lvclass">, "IProperty out"=w220:refnum<class "IProperty.lvclass">)  [unwired: 6 in, 1 out]
                        n88 = call <instrlib>:"getItemType.vi"("error in (no error)"=w219, "IProperty in"=w220) -> ("error out"=w215:errorcluster, "Item Type out"=w217:T8)  [unwired: 7 in, 1 out]
                        n89 = call <instrlib>:"CoreTypeToString.vi"("Value Type out"=w217) -> ("String"=w216:string)  [unwired: 4 in]
                        n90 = case shown="\"ctString\"" w216 {
                          tunnel: w218 -> [_ w230 w237 w243]
                          tunnel: w215 -> [w223 w229 w236 w242]
                          tunnel: [_ w228 w235 w238] -> w211
                          tunnel: [w223 w226 w233 w240] -> w214
                          frame Default {
                          }
                          frame "ctInt" {
                            n91 = call-poly <instrlib>:"_borrowInterface.vi"("error in (no error)"=w229, "IBaseObject in"=w230) -> ("error out"=w227:errorcluster, "Dict out"=w225:refnum<class "IDict.lvclass">)  [unwired: 6 in, 2 out]
                            n92 = call-poly <instrlib>:"_getValueList.vi"("error in (no error)"=w227, "IDict in"=w225) -> ("error out"=w226:errorcluster, "Integer Value list out"=w224:i32[])  [unwired: 7 in, 1 out]
                            n93 = Number To Decimal String(number=w224) -> (decimal integer string=w228:string[])  [unwired: 1 in]
                          }
                          frame "ctFloat" {
                            n94 = call-poly <instrlib>:"_borrowInterface.vi"("error in (no error)"=w236, "IBaseObject in"=w237) -> ("error out"=w234:errorcluster, "Dict out"=w232:refnum<class "IDict.lvclass">)  [unwired: 6 in, 2 out]
                            n95 = call-poly <instrlib>:"_getValueList.vi"("error in (no error)"=w234, "IDict in"=w232) -> ("error out"=w233:errorcluster, "Integer Value list out"=w231:dbl[])  [unwired: 7 in, 1 out]
                            n96 = Number To Decimal String(number=w231) -> (decimal integer string=w235:string[])  [unwired: 1 in]
                          }
                          frame "ctString" {
                            n97 = call-poly <instrlib>:"_borrowInterface.vi"("error in (no error)"=w242, "IBaseObject in"=w243) -> ("error out"=w241:errorcluster, "Dict out"=w239:refnum<class "IDict.lvclass">)  [unwired: 6 in, 2 out]
                            n98 = call-poly <instrlib>:"_getValueList.vi"("error in (no error)"=w241, "IDict in"=w239) -> ("error out"=w240:errorcluster, "String Value list out"=w238:string[])  [unwired: 7 in, 1 out]
                          }
                        }
                        n99 = Index Array(array=w211) -> (element=w212:string)  [unwired: 1 in]
                        n100 = property on="Selection Values" class="CmbBox"("Strings[]"=w211, "Visible"=TRUE, "Value"=w212) -> ()  [unwired: 2 in, 2 out]
                      }
                    }
                  }
                  frame True {
                    n101 = property on="Selection Values" class="CmbBox"("Strings And Values[]"=T5 [] ("Strings And Values []"), "Visible"=FALSE) -> ()  [unwired: 2 in, 2 out]
                  }
                }
                n102 = Bundle By Name(cluster=w170, "Selected.Property"=w169) -> (w166:T2)
                n103 = Not(x=w168) -> (.not. x?=w171:bool)
              }
              frame True {
                n104 = invoke class="Tree (strict)" method="Navigate Tree.Get Parent"(reference=w254, "tag"=w253) -> ("Navigate Tree:Get Parent"=w256:string)  [unwired: 2 in, 3 out]
                n105 = Look In Map(map=w255, key=w256) -> (key not found?=w252:bool, value=w251:refnum<class "IProperty.lvclass">)  [unwired: 1 in]
                n106 = case shown="False" w252 {
                  tunnel: w251 -> [w266 _]
                  tunnel: w257 -> [w265 w273]
                  tunnel: w250 -> [w262 w275]
                  tunnel: [w260 w275] -> w249
                  tunnel: [w259 TRUE] -> w248
                  tunnel: [w258 w273] -> w247
                  frame False {
                    n107 = call <instrlib>:"getPropertyType.vi"("error in (no error)"=w265, "IProperty in"=w266) -> ("error out"=w258:errorcluster, "Property Type out"=w264:T9, "IProperty out"=w261:refnum<class "IProperty.lvclass">)  [unwired: 7 in]
                    n108 = call <instrlib>:"PropertyTypeToString.vi"("Property Type"=w264) -> ("String"=w263:string)  [unwired: 4 in]
                    n109 = case shown="\"List\"" w263 {
                      tunnel: w262 -> [w268 w272]
                      tunnel: w261 -> [_ w271]
                      tunnel: [w268 w270] -> w260
                      tunnel: [TRUE FALSE] -> w259
                      frame Default {
                      }
                      frame "List" {
                        n110 = Bundle By Name(cluster=w272, "Selected.Property"=w271) -> (w270:T2)
                      }
                    }
                  }
                  frame True {
                  }
                }
              }
            }
            n111 = Or(x=w156, y=w155) -> (x .or. y?=w154:bool)
            n112 = event-data("Discard?"=w154) -> ()  [unwired: 1 in, 1 out]
          }
          event "Tree.Properties": Edit Cell {
            n113 = event-data() -> ("String"=w277:string, "CtlRef"=w278:refnum<vi>, "Tag"=w279:string)  [unwired: 1 in]
            n114 = Unbundle By Name(w289) -> ("Selected.Property"=w284:refnum<class "IProperty.lvclass">)
            n115 = call <instrlib>:"getPropertyType.vi"("error in (no error)"=w280, "IProperty in"=w284) -> ("error out"=w283:errorcluster, "Property Type out"=w281:T9, "IProperty out"=w276:refnum<class "IProperty.lvclass">)  [unwired: 7 in]
            n116 = call <instrlib>:"PropertyTypeToString.vi"("Property Type"=w281) -> ("String"=w282:string)  [unwired: 4 in]
            n117 = case shown="\"List\"" w282 {
              tunnel: w283 -> [w290 w296 w301 w304 w312 w323 w330]
              tunnel: [w290 w292 w297 w303 w311 w322 w324] -> w286
              tunnel: w277 -> [_ w295 w300 w308 w309 w320 _]
              tunnel: [_ w293 w298 w302 w310 w321 w325] -> w285
              tunnel: w279 -> [_ _ _ _ _ _ w332]
              tunnel: w278 -> [_ _ _ _ _ _ w331]
              frame Default {
                n118 = One Button Dialog(message="Data type not supported yet!") -> ()  [unwired: 1 in, 1 out]
              }
              frame "Float" {
                n119 = Fract/Exp String To Number(string=w295) -> (number=w294:dbl)  [unwired: 3 in, 1 out]
                n120 = call <instrlib>:"createFloat.vi"("error in (no error)"=w296, "Value"=w294) -> ("error out"=w292:errorcluster, "IInteger out"=w293:refnum<class "IFloat.lvclass">)  [unwired: 8 in]
              }
              frame "Int" {
                n121 = Decimal String To Number(string=w300) -> (number=w299:i32)  [unwired: 2 in, 1 out]
                n122 = call <instrlib>:"createInteger.vi"("error in (no error)"=w301, "Value"=w299) -> ("error out"=w297:errorcluster, "IInteger out"=w298:refnum<class "IInteger.lvclass">)  [unwired: 8 in]
              }
              frame "Bool" {
                n123 = Match True/False String(2:"No" ("false string"), 3:"Yes" ("true string"), 4:w308) -> (0:w305:bool)  [unwired: 1 out]
                n124 = call <instrlib>:"createBoolean.vi"("error in (no error)"=w304, "bool"=w305) -> ("error out"=w303:errorcluster, "IBoolean out"=w302:refnum<class "IBoolean.lvclass">)  [unwired: 8 in]
              }
              frame "String" {
                n125 = call <instrlib>:"createString.vi"("error in (no error)"=w312, "String"=w309) -> ("error out"=w311:errorcluster, "IString out"=w310:refnum<class "IString.lvclass">)  [unwired: 8 in]
              }
              frame "Ratio" {
                n126 = Search/Split String(string=w320, search string/char (-)="/") -> (substring before match=w318:string, match + rest of string=w317:string)  [unwired: 1 in, 1 out]
                n127 = call <vilib>:"Trim Whitespace.vi"("string"=w318) -> ("trimmed string"=w316:string)  [unwired: 1 in]
                n128 = call <vilib>:"Trim Whitespace.vi"("string"=w317) -> ("trimmed string"=w314:string)  [unwired: 1 in]
                n129 = Decimal String To Number(string=w316) -> (number=w315:i32)  [unwired: 2 in, 1 out]
                n130 = Decimal String To Number(string=w314) -> (number=w313:i32)  [unwired: 2 in, 1 out]
                n131 = call <instrlib>:"createRatio.vi"("error in (no error)"=w323, "Denominator"=w313, "Numerator"=w315) -> ("error out"=w322:errorcluster, "IRatio out"=w321:refnum<class "IRatio.lvclass">)  [unwired: 7 in]
              }
              frame "List" {
                n132 = call <instrlib>:"getAllChildren.vi"("error in (no error)"=w330, "Child Tag in"=w332, "Tree ref in"=w331) -> ("error out"=w333:errorcluster, "Values"=w328:string[], "Value Type"=w329:string)  [unwired: 4 in, 2 out]
                n133 = call <instrlib>:"createList.vi"("error in (no error)"=w333) -> ("error out"=w326:errorcluster, "IList out"=w327:refnum<class "IList.lvclass">)  [unwired: 9 in]
                n134 = case shown="Default" w329 {
                  tunnel: w328 -> [_ w340 w353 w366 w381]
                  tunnel: w327 -> [_ w339 w352 w365 w380]
                  tunnel: w326 -> [w335 w338 w351 w364 w379]
                  tunnel: [_ w336 w349 w362 w377] -> w325
                  tunnel: [w335 w337 w350 w363 w378] -> w324
                  frame Default {
                    n135 = One Button Dialog(message="Data type of list not supported yet!") -> ()  [unwired: 1 in, 1 out]
                  }
                  frame "ctFloat" {
                    n136 = for {
                      tunnel: w340 -> [w346] mode=indexing
                      shift-right: [w343] -> w336
                      shift-left: w339 -> [w344]
                      shift-right: [w342] -> w337
                      shift-left: w338 -> [w347]
                      n137 = Fract/Exp String To Number(string=w346) -> (number=w345:dbl)  [unwired: 3 in, 1 out]
                      n138 = call <instrlib>:"createFloat.vi"("error in (no error)"=w347, "Value"=w345) -> ("error out"=w348:errorcluster, "IInteger out"=w341:refnum<class "IFloat.lvclass">)  [unwired: 8 in]
                      n139 = call <instrlib>:"pushBack.vi"("error in (no error)"=w348, "Object in"=w341, "IList in"=w344) -> ("error out"=w342:errorcluster, "IList out"=w343:refnum<class "IList.lvclass">)  [unwired: 6 in, 1 out]
                    }
                  }
                  frame "ctInt" {
                    n140 = for {
                      tunnel: w353 -> [w359] mode=indexing
                      shift-right: [w356] -> w349
                      shift-left: w352 -> [w357]
                      shift-right: [w355] -> w350
                      shift-left: w351 -> [w360]
                      n141 = Decimal String To Number(string=w359) -> (number=w358:i32)  [unwired: 2 in, 1 out]
                      n142 = call <instrlib>:"createInteger.vi"("error in (no error)"=w360, "Value"=w358) -> ("error out"=w361:errorcluster, "IInteger out"=w354:refnum<class "IInteger.lvclass">)  [unwired: 8 in]
                      n143 = call <instrlib>:"pushBack.vi"("error in (no error)"=w361, "Object in"=w354, "IList in"=w357) -> ("error out"=w355:errorcluster, "IList out"=w356:refnum<class "IList.lvclass">)  [unwired: 6 in, 1 out]
                    }
                  }
                  frame "ctBool" {
                    n144 = for {
                      tunnel: w366 -> [w368] mode=indexing
                      shift-right: [w371] -> w362
                      shift-left: w365 -> [w372]
                      shift-right: [w370] -> w363
                      shift-left: w364 -> [w373]
                      n145 = case shown="Default" w368 {
                        tunnel: [FALSE TRUE] -> w367
                        frame Default {
                        }
                        frame "Yes" {
                        }
                      }
                      n146 = call <instrlib>:"createBoolean.vi"("error in (no error)"=w373, "bool"=w367) -> ("error out"=w374:errorcluster, "IBoolean out"=w369:refnum<class "IBoolean.lvclass">)  [unwired: 8 in]
                      n147 = call <instrlib>:"pushBack.vi"("error in (no error)"=w374, "Object in"=w369, "IList in"=w372) -> ("error out"=w370:errorcluster, "IList out"=w371:refnum<class "IList.lvclass">)  [unwired: 6 in, 1 out]
                    }
                  }
                  frame "ctString" {
                    n148 = for {
                      tunnel: w381 -> [w382] mode=indexing
                      shift-right: [w385] -> w377
                      shift-left: w380 -> [w386]
                      shift-right: [w384] -> w378
                      shift-left: w379 -> [w387]
                      n149 = call <instrlib>:"createString.vi"("error in (no error)"=w387, "String"=w382) -> ("error out"=w388:errorcluster, "IString out"=w383:refnum<class "IString.lvclass">)  [unwired: 8 in]
                      n150 = call <instrlib>:"pushBack.vi"("error in (no error)"=w388, "Object in"=w383, "IList in"=w386) -> ("error out"=w384:errorcluster, "IList out"=w385:refnum<class "IList.lvclass">)  [unwired: 6 in, 1 out]
                    }
                  }
                }
              }
            }
            n151 = call <instrlib>:"setValue.vi"("error in (no error)"=w286, "Value in"=w285, "IProperty in"=w276) -> ("error out"=w287:errorcluster)  [unwired: 7 in, 1 out]
          }
          event "Selection Values": Value Change {
            # "Test-purpose"
            n152 = event-data() -> ("NewVal"=w391:string)  [unwired: 1 in]
            n153 = Unbundle By Name(w392) -> ("Selected.Property"=w393:refnum<class "IProperty.lvclass">)
            n154 = call <instrlib>:"getSelectionValuesLength.vi"("IProperty in"=w393) -> ("Selection Values Null?"=w394:bool, "List?"=w396:bool)  [unwired: 5 in, 4 out]
            n155 = case shown="False" w394 {
              tunnel: [w399 w495] -> w389
              tunnel: w393 -> [w397 _]
              tunnel: w395 -> [w401 w495]
              tunnel: w396 -> [w400 _]
              tunnel: w391 -> [w398 _]
              frame False {
                n156 = case shown="False" w400 {
                  tunnel: w397 -> [w418 w471]
                  tunnel: w401 -> [w417 w470]
                  tunnel: [w411 w463] -> w399
                  tunnel: w398 -> [w413 _]
                  tunnel: w397 -> [w409 _]
                  frame True {
                    # "List"
                    n157 = call <instrlib>:"getSelectionValues.vi"("error in (no error)"=w417, "IProperty in"=w418) -> ("error out"=w407:errorcluster, "Selection Values out"=w416:refnum<class "IBaseObject.lvclass">, "IProperty out"=w408:refnum<class "IProperty.lvclass">)  [unwired: 6 in, 1 out]
                    n158 = call <instrlib>:"getItemType.vi"("error in (no error)"=w407, "IProperty in"=w408) -> ("error out"=w405:errorcluster, "Item Type out"=w415:T8)  [unwired: 7 in, 1 out]
                    n159 = call <instrlib>:"getValueType.vi"("error in (no error)"=w407, "IProperty in"=w408) -> ("error out"=w404:errorcluster, "Value Type out"=w403:T8)  [unwired: 7 in, 1 out]
                    n160 = call <instrlib>:"CoreTypeToString.vi"("Value Type out"=w415) -> ("String"=w414:string)  [unwired: 4 in]
                    n161 = Merge Errors(w405, w404) -> (w406:errorcluster)
                    n162 = call <instrlib>:"CoreTypeToString.vi"("Value Type out"=w403) -> ("String"=w402:string)  [unwired: 4 in]
                    n163 = case shown="\"ctString\"" w414 {
                      tunnel: w416 -> [_ w427 w448 w457]
                      tunnel: w406 -> [w419 w426 w447 w456]
                      tunnel: [w419 w424 w443 w453] -> w412
                      tunnel: w413 -> [_ w423 w446 w455]
                      tunnel: [_ w422 w441 w452] -> w410
                      tunnel: w402 -> [_ w421 _ _]
                      frame Default {
                      }
                      frame "ctString" {
                        n164 = call-poly <instrlib>:"_borrowInterface.vi"("error in (no error)"=w426, "IBaseObject in"=w427) -> ("error out"=w428:errorcluster, "List out"=w429:refnum<class "IList.lvclass">)  [unwired: 6 in, 2 out]
                        n165 = call-poly <instrlib>:"_getList.vi"("error in (no error)"=w428, "IList in"=w429) -> ("error out"=w425:errorcluster, "String List out"=w420:string[])  [unwired: 8 in]
                        n166 = case shown="\"ctString\"" w421 {
                          tunnel: w425 -> [w430 w434 w436]
                          tunnel: [w430 w433 w437] -> w424
                          tunnel: w423 -> [_ w432 w439]
                          tunnel: [_ w431 w435] -> w422
                          tunnel: w420 -> [_ _ w440]
                          frame Default {
                          }
                          frame "ctString" {
                            n167 = call <instrlib>:"createString.vi"("error in (no error)"=w434, "String"=w432) -> ("error out"=w433:errorcluster, "IString out"=w431:refnum<class "IString.lvclass">)  [unwired: 8 in]
                          }
                          frame "ctInt" {
                            n168 = Search 1D Array(1D array=w440, element=w439) -> (index of element=w438:i32)  [unwired: 1 in]
                            n169 = call <instrlib>:"createInteger.vi"("error in (no error)"=w436, "Value"=w438) -> ("error out"=w437:errorcluster, "IInteger out"=w435:refnum<class "IInteger.lvclass">)  [unwired: 8 in]
                          }
                        }
                      }
                      frame "ctFloat" {
                        n170 = call-poly <instrlib>:"_borrowInterface.vi"("error in (no error)"=w447, "IBaseObject in"=w448) -> ("error out"=w449:errorcluster, "List out"=w450:refnum<class "IList.lvclass">)  [unwired: 6 in, 2 out]
                        n171 = call-poly <instrlib>:"_getList.vi"("error in (no error)"=w449, "IList in"=w450) -> ("error out"=w442:errorcluster)  [unwired: 8 in, 1 out]
                        n172 = Fract/Exp String To Number(use system decimal point (T)=FALSE, string=w446) -> (number=w444:dbl)  [unwired: 2 in, 1 out]
                        n173 = call <instrlib>:"createFloat.vi"("error in (no error)"=w442, "Value"=w444) -> ("error out"=w443:errorcluster, "IInteger out"=w441:refnum<class "IFloat.lvclass">)  [unwired: 8 in]
                      }
                      frame "ctInt" {
                        n174 = call-poly <instrlib>:"_borrowInterface.vi"("error in (no error)"=w456, "IBaseObject in"=w457) -> ("error out"=w458:errorcluster, "List out"=w459:refnum<class "IList.lvclass">)  [unwired: 6 in, 2 out]
                        n175 = call-poly <instrlib>:"_getList.vi"("error in (no error)"=w458, "IList in"=w459) -> ("error out"=w454:errorcluster)  [unwired: 8 in, 1 out]
                        n176 = Decimal String To Number(string=w455) -> (number=w451:i32)  [unwired: 2 in, 1 out]
                        n177 = call <instrlib>:"createInteger.vi"("error in (no error)"=w454, "Value"=w451) -> ("error out"=w453:errorcluster, "IInteger out"=w452:refnum<class "IInteger.lvclass">)  [unwired: 8 in]
                      }
                    }
                    n178 = call <instrlib>:"setValue.vi"("error in (no error)"=w412, "Value in"=w410, "IProperty in"=w409) -> ("error out"=w411:errorcluster)  [unwired: 7 in, 1 out]
                  }
                  frame False {
                    # "Dict"
                    n179 = call <instrlib>:"getSelectionValues.vi"("error in (no error)"=w470, "IProperty in"=w471) -> ("error out"=w468:errorcluster, "Selection Values out"=w467:refnum<class "IBaseObject.lvclass">, "IProperty out"=w469:refnum<class "IProperty.lvclass">)  [unwired: 6 in, 1 out]
                    n180 = call <instrlib>:"getItemType.vi"("error in (no error)"=w468, "IProperty in"=w469) -> ("error out"=w464:errorcluster, "Item Type out"=w466:T8)  [unwired: 7 in, 1 out]
                    n181 = call <instrlib>:"CoreTypeToString.vi"("Value Type out"=w466) -> ("String"=w465:string)  [unwired: 4 in]
                    n182 = case shown="\"ctInt\"" w465 {
                      tunnel: w467 -> [_ w479 w486 w492]
                      tunnel: w464 -> [w472 w478 w485 w491]
                      tunnel: [_ w477 w484 w487] -> w460
                      tunnel: [w472 w475 w482 w489] -> w463
                      frame Default {
                      }
                      frame "ctInt" {
                        n183 = call-poly <instrlib>:"_borrowInterface.vi"("error in (no error)"=w478, "IBaseObject in"=w479) -> ("error out"=w476:errorcluster, "Dict out"=w474:refnum<class "IDict.lvclass">)  [unwired: 6 in, 2 out]
                        n184 = call-poly <instrlib>:"_getValueList.vi"("error in (no error)"=w476, "IDict in"=w474) -> ("error out"=w475:errorcluster, "Integer Value list out"=w473:i32[])  [unwired: 7 in, 1 out]
                        n185 = Number To Decimal String(number=w473) -> (decimal integer string=w477:string[])  [unwired: 1 in]
                      }
                      frame "ctFloat" {
                        n186 = call-poly <instrlib>:"_borrowInterface.vi"("error in (no error)"=w485, "IBaseObject in"=w486) -> ("error out"=w483:errorcluster, "Dict out"=w481:refnum<class "IDict.lvclass">)  [unwired: 6 in, 2 out]
                        n187 = call-poly <instrlib>:"_getValueList.vi"("error in (no error)"=w483, "IDict in"=w481) -> ("error out"=w482:errorcluster, "Integer Value list out"=w480:dbl[])  [unwired: 7 in, 1 out]
                        n188 = Number To Decimal String(number=w480) -> (decimal integer string=w484:string[])  [unwired: 1 in]
                      }
                      frame "ctString" {
                        n189 = call-poly <instrlib>:"_borrowInterface.vi"("error in (no error)"=w491, "IBaseObject in"=w492) -> ("error out"=w490:errorcluster, "Dict out"=w488:refnum<class "IDict.lvclass">)  [unwired: 6 in, 2 out]
                        n190 = call-poly <instrlib>:"_getValueList.vi"("error in (no error)"=w490, "IDict in"=w488) -> ("error out"=w489:errorcluster, "String Value list out"=w487:string[])  [unwired: 7 in, 1 out]
                      }
                    }
                    n191 = Index Array(array=w460) -> (element=w461:string)  [unwired: 1 in]
                    n192 = property on="Selection Values" class="CmbBox"("Strings[]"=w460, "Visible"=TRUE, "Value"=w461) -> ()  [unwired: 2 in, 2 out]
                  }
                }
              }
              frame True {
                n193 = property on="Selection Values" class="CmbBox"("Strings And Values[]"=T5 [] ("Strings And Values []"), "Visible"=FALSE) -> ()  [unwired: 2 in, 2 out]
              }
            }
          }
          event "btn:PropertyRefresh": Value Change {
            # "Test-purpose"
            n194 = event-data() -> ()  [unwired: 1 in, 6 out]
            n195 = property on="btn:PropertyRefresh" class="Bool (strict)"("Value"=FALSE ("btn:PropertyRefresh")) -> ()  [unwired: 2 in, 2 out]
          }
        }
      }
      frame "- PROPERTIES.traverse" {
        n196 = control-ref of="This VI"() -> (w508:refnum<vi>)
        n197 = property class="VI"(reference=w508, error in=w517) -> (error out=w505:errorcluster, "Panel"=w507:refnum<vi>)  [unwired: 1 out]
        n198 = property class="Pnl"(reference=w507, error in=w505, "DeferPanUpdts"=TRUE ("Defer Panel Updates")) -> (reference out=w515:refnum<vi>, error out=w501:errorcluster)
        n199 = invoke on="Tree.Properties" class="Tree (strict)" method="Edit Tree Items.Delete"(error in=w501) -> (error out=w500:errorcluster)  [unwired: 4 in, 4 out]
        n200 = Unbundle By Name(w513) -> ("Selected.Node"=w512:refnum<class "IComponent.lvclass">)
        n201 = call <instrlib>:"treeTraverseComponentPropertiesRecursive.vi"("error in (no error)"=w500, "IPropertyObject in"=w512, "Context in"=w513) -> ("error out"=w514:errorcluster, "Context out"=w510:T2)  [unwired: 6 in, 1 out]
        n202 = call <instrlib>:"markReadOnly.vi"("error in (no error)"=w514, "Context in"=w510) -> ("error out"=w509:errorcluster, "Context out"=w511:T2)  [unwired: 8 in]
        n203 = property class="Pnl"(reference=w515, error in=w509, "DeferPanUpdts"=FALSE ("Defer Panel Updates")) -> (reference out=w503:refnum<vi>, error out=w502:errorcluster)
        n204 = Close Reference(reference=w503, error in (no error)=w502) -> (error out=w516:errorcluster)
      }
      frame "STOP" {
        # "Remove instance"
        n205 = Unbundle By Name(w534) -> ("Simulator.Instance"=w533:refnum<class "IComponent.lvclass">, "Instance"=w532:refnum<class "IComponent.lvclass">, "Simulator"=w531:refnum<class "IComponent.lvclass">, "Nodes"=w530:map{string, refnum<class "IComponent.lvclass">}, "Properties"=w529:map{string, refnum<class "IProperty.lvclass">})
        n206 = for {
          tunnel: [w542] -> w526 mode=indexing
          tunnel: w530 -> [w543] mode=indexing
          n207 = Unbundle By Name(w543) -> ("Node"=w542:refnum<class "IComponent.lvclass">)
        }
        n208 = for {
          tunnel: [w540] -> w528 mode=indexing
          tunnel: w529 -> [w541] mode=indexing
          n209 = Unbundle By Name(w541) -> ("Property"=w540:refnum<class "IProperty.lvclass">)
        }
        n210 = Delete From Array(array=w526, index=0) -> (array with subset deleted=w525:refnum<class "IComponent.lvclass">[])  [unwired: 1 in, 1 out]
        n211 = call <instrlib>:"releaseRefArray.vi"("IBaseObject in"=w528) -> ("error out"=w520:errorcluster)  [unwired: 10 in]
        n212 = call <instrlib>:"releaseRefArray.vi"("error in (no error)"=w520, "IBaseObject in"=w525) -> ("error out"=w521:errorcluster)  [unwired: 9 in]
        n213 = call-dynamic "releaseRef.vi"("error in (no error)"=w521, "IBaseObject in"=w531) -> ("error out"=w523:errorcluster)  [unwired: 9 in]
        n214 = call-dynamic "releaseRef.vi"("error in (no error)"=w523, "IBaseObject in"=w532) -> ("error out"=w522:errorcluster)  [unwired: 9 in]
        n215 = call-dynamic "releaseRef.vi"("error in (no error)"=w522, "IBaseObject in"=w533) -> ("error out"=w519:errorcluster)  [unwired: 9 in]
        n216 = case shown="True" w527 {
          tunnel: w519 -> [_ w538]
          frame False {
          }
          frame True {
            n217 = control-ref of="This VI"() -> (w539:refnum<vi>)
            n218 = invoke class="VI" method="FP.Close"(reference=w539, error in=w538) -> ()  [unwired: 1 in, 3 out]
          }
        }
      }
      frame "ERROR" {
        n219 = call <vilib>:"Simple Error Handler.vi"("error in (no error)"=w547) -> ("error out"=w548:errorcluster)  [unwired: 4 in, 4 out]
        n220 = call <vilib>:"Clear Errors.vi"("error in (no error)"=w548) -> ("error out"=w546:errorcluster)  [unwired: 5 in, 1 out]
      }
    }
    n221 = Select(t=State."ERROR" ("Enum"), s=w18, f=w13) -> (s? t:f=w15:T4)
  }
  "error out" <- w2
